vi "Final Line Detection System_2.vi"() -> ()   [LabVIEW 2017]
uses:
  <vilib>/userdefined/High Color/IMAQdx.ctl
  <vilib>/vision/driver/NI_Vision_Acquisition_Software.lvlib
  <vilib>/vision/NI_Vision_Development_Module.lvlib
panel:
  in  "Line Colour":string(combo)="Black"
  out "String 2":string
  in  "Maintenance":bool
  out "SpeechLib.ISpeechVoice 2":refnum<k7>
  in  "CHOOSE A VOICE:":i32(ring) items=["Microsoft Hazel Desktop - English (Great Britain)", "eSpeak-EN+M2", "eSpeak-EN-N"]
  in  "SpeechLib.ISpeechVoice":refnum<k7>
  out "Caution":bool
  out "Warning Message":string="Warning Obstacle!"
  out "Front IR Output voltage":dbl
  out "Back IR Output voltage":dbl
  out "Right IR Output voltage":dbl
  in  "Back IR Object Distance":dbl(knob)=80.0 min=0.0 max=100.0 step=1.0 scale=10.0..80.0
  in  "Front IR Object Distance":dbl(knob)=80.0 min=0.0 max=100.0 step=1.0 scale=10.0..80.0
  in  "Right IR Object Distance":dbl(knob)=80.0 min=0.0 max=100.0 step=1.0 scale=10.0..80.0
  out "error out 2":errorcluster
  out "Video Stream":T1(plugin-control)
  in  "stop":bool
  out "Found":bool
  out "error out 3":errorcluster
  out "error out 8":errorcluster
  out "error out 4":errorcluster
  in  "Barcode Types To Search":u32[](array[ring])=[6, 4] items=["Reserved", "Codabar", "Code 39", "Code 93", "Code 128", "EAN 8", "EAN 13", "Interleaved 2 of 5", "MSI", "UPCA", "Pharmacode", "RSS Limited"]
  out "error out 5":errorcluster
  in  "Select Vision System":string(combo)="None"
  out "Data":string
  in  "Recipients":string="chyslop@hotmail.co.uk, b8026896@my.shu.ac.uk,"
  in  "Subject":string
  in  "Message":string
  out "Primary IP Address":string
  out "All Other IP Addresses":string
  out "Number of Addresses":i32
  out "error out":errorcluster
  in  "Send":bool
  out "String":string
  in  "Session In":T2="cam1"
  in  "Noise IR Sensor 0 = no noise":dbl
  out "Left IR Output voltage":dbl
  in  "Left IR Object Distance":dbl(knob)=80.0 min=0.0 max=100.0 step=1.0 scale=10.0..80.0
  out "Right Motor Speedometer (m/s)":dbl(knob) scale=-2.5..2.5
  out "Left Motor Speedometer (m/s)":dbl(knob) scale=-2.5..2.5
  out "Right voltage more than 0?":bool
  out "Right Line sensor output voltage":dbl
  in  "Right Line Detector Sensor":dbl(slide) scale=0.0..5.0
  out "Left Voltage more than 0?":bool
  out "Left Line sensor output voltage":dbl
  in  "Left Line Detector Sensor":dbl(slide) scale=0.0..5.0
  out "Middle voltage more than 0?":bool
  out "Middle Line sensor output voltage":dbl
  in  "Middle Line Detector Sensor":dbl(slide) scale=0.0..5.0
  in  "Noise Line sensor, 0 = no noise":dbl
  in  "Stop":bool
  out "Direction":string
  out "Speedometer (m/s)":dbl(knob) scale=0.0..3.0
  in  "% Power":dbl(slide) scale=0.0..100.0
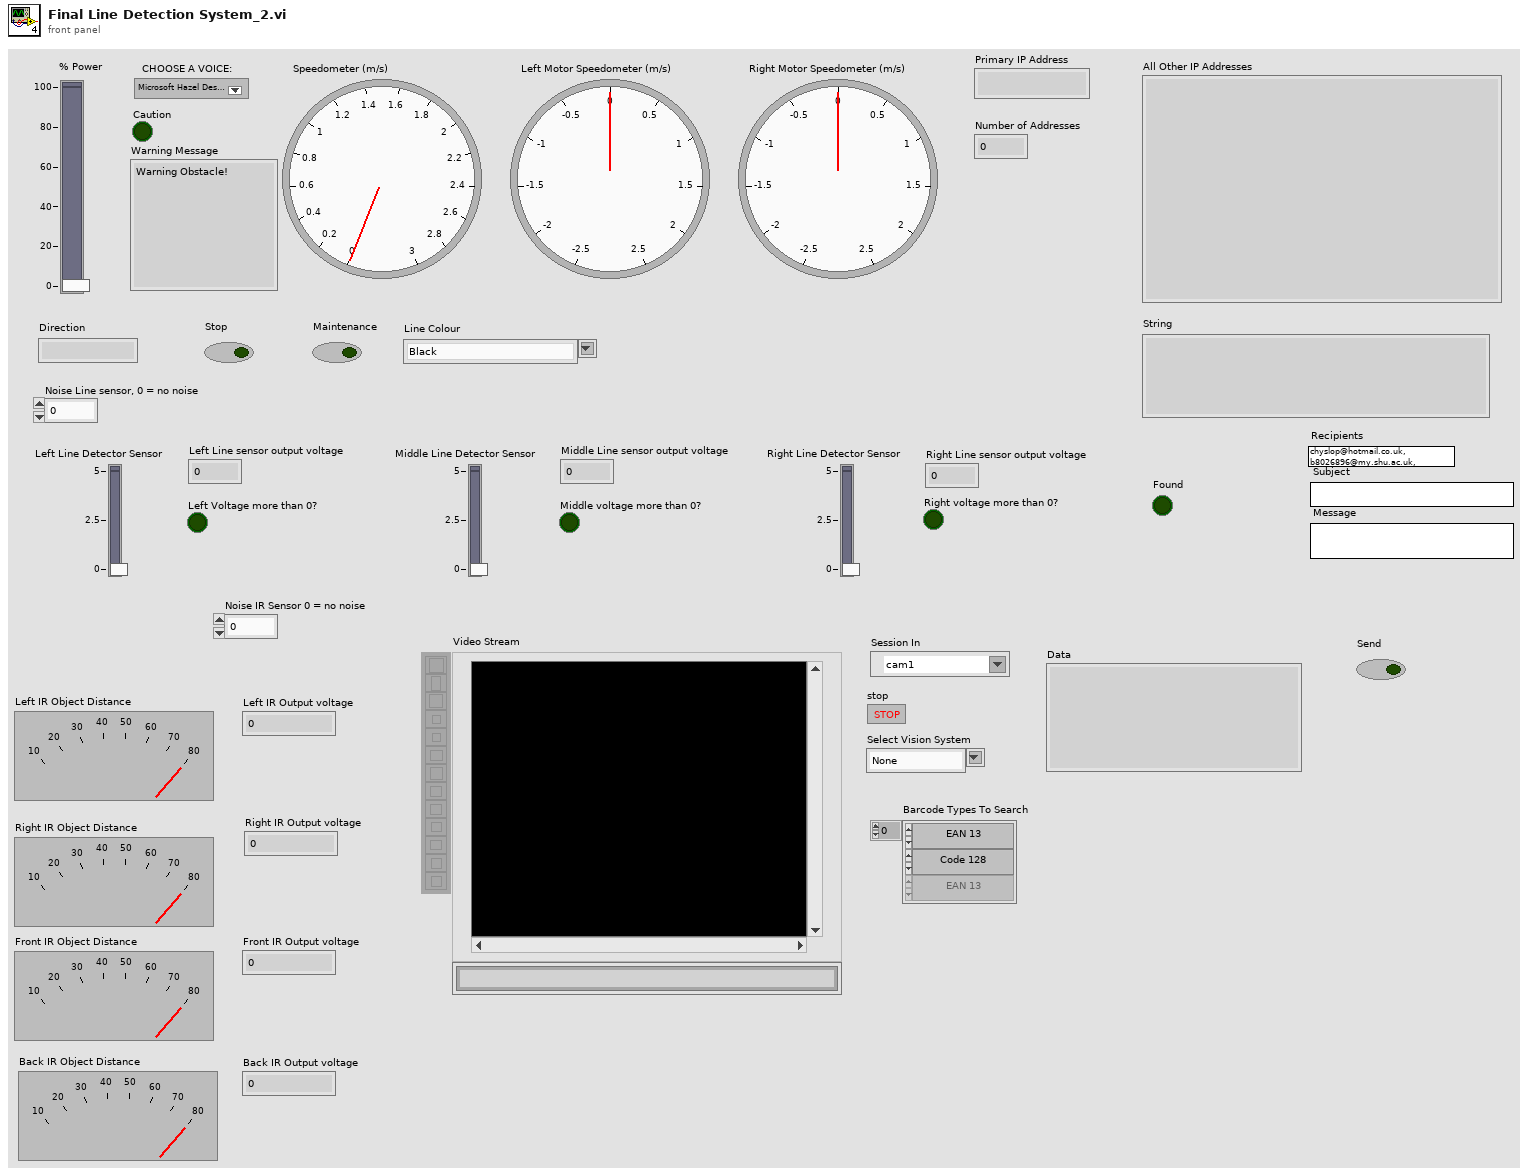
[diagram p1: front panel]
types:
  T1 = typedef "IMAQ Image.ctl" = refnum<image>
  T2 = typedef "IMAQdx.ctl" = refnum<k21>
  T3 = typedef "Image Type" = u32
  T4 = cluster{"Data":string, "Special Char 1":string, "Special Char 2":string, "Checksum(s)":string, "Barcode Type":u32, "Confidence Level":sgl, "Bounding Box":cluster{"x":sgl, "y":sgl}[]}[]
  T5 = cluster{"Data":string, "Special Char 1":string, "Special Char 2":string, "Checksum(s)":string, "Barcode Type":u32, "Confidence Level":sgl, "Bounding Box":cluster{"x":sgl, "y":sgl}[]}
  T6 = typedef "QR Code Report.ctl" = cluster{"Found?":bool, "Data":string, "Bounding Box":cluster{"x":sgl, "y":sgl}[], "Errors Corrected":u32, "Dimensions (Rows/Cols)":u32, "Version":u32, "QR Model":T7, "Stream Mode":T8, "Barcode Polarity":T9, "Mirrored?":bool, "Append Stream Position":u32, "Size of Append Stream":u32, "First EAN-128 ID":i32, "First Alternate Language ID":i32, "Append Stream ID":u32, "Minimum Edge Strength":u32, "Demodulation Mode":T10, "Cell Sample Size":T11, "Cell Filter Mode":T12}
  T7 = typedef "QR Code Model Type.ctl" = i32
  T8 = typedef "QR Code Stream Mode Type.ctl" = i32
  T9 = typedef "Data Matrix Polarity.ctl" = i32
  T10 = typedef "Demodulation Mode.ctl" = i32
  T11 = typedef "Cell Sample Size.ctl" = i32
  T12 = typedef "Cell Filter Mode.ctl" = i32
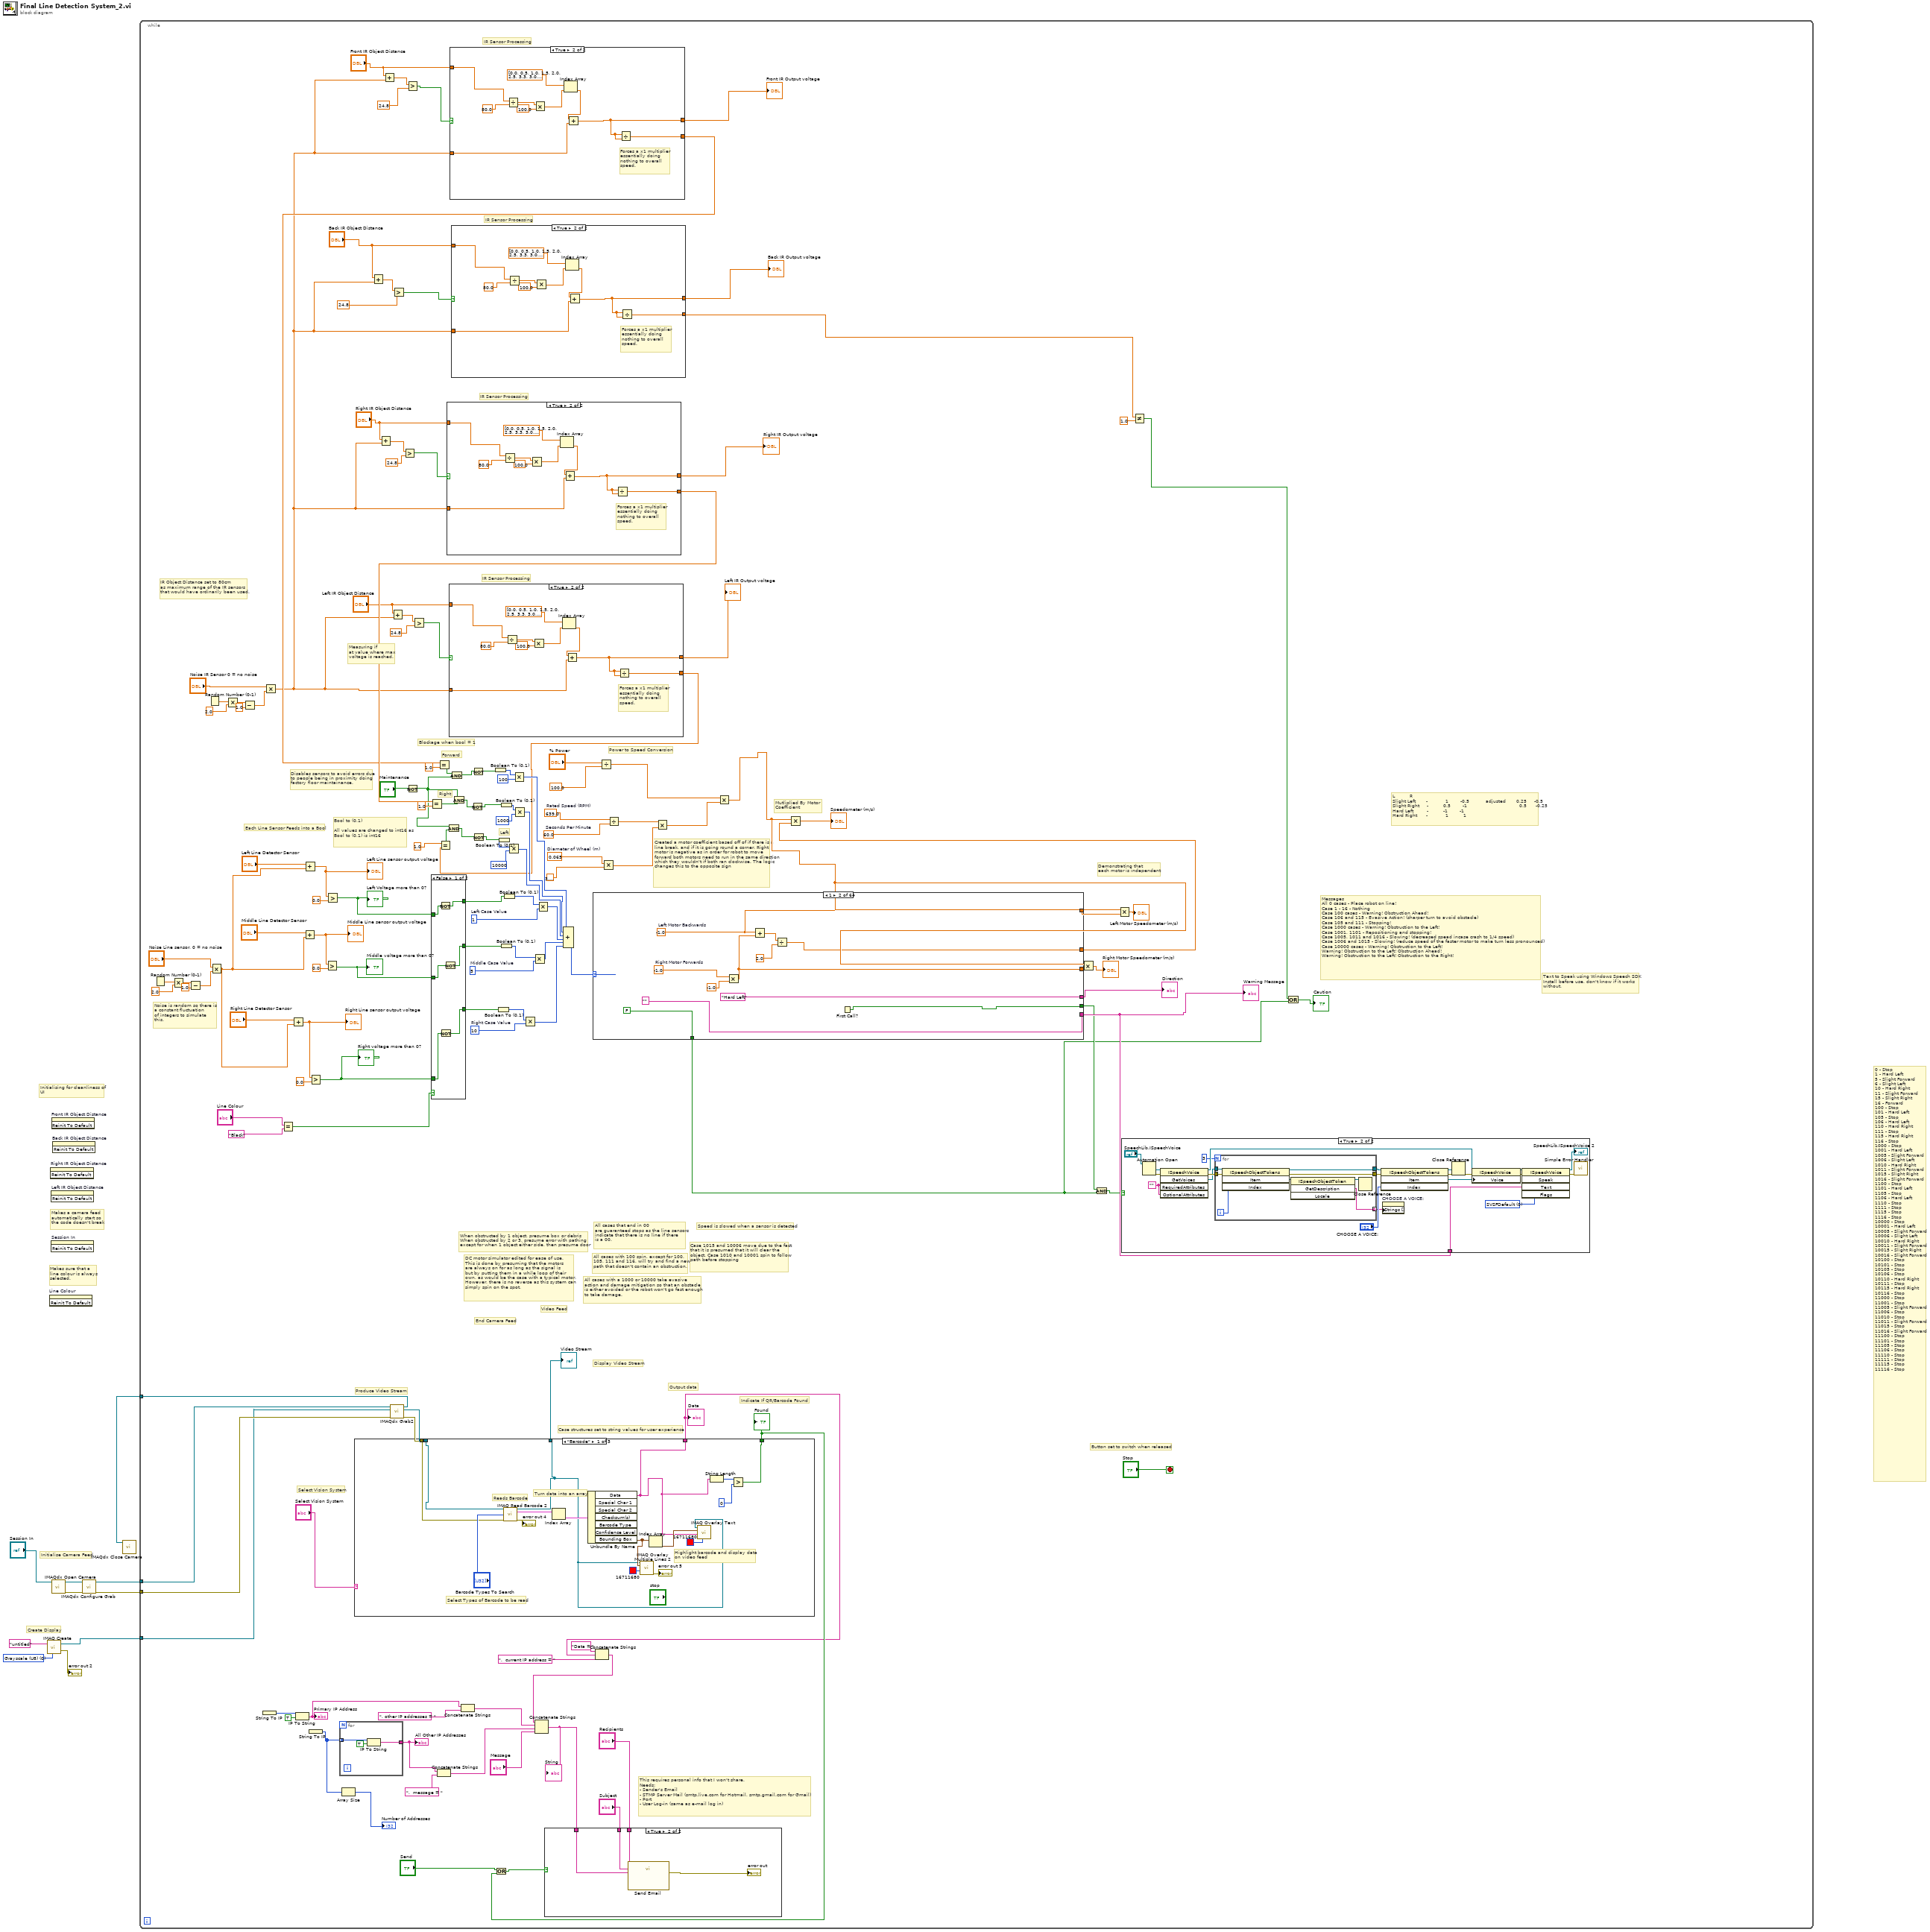
[diagram p0: block diagram]
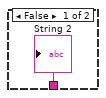
[diagram p3: hidden frame]
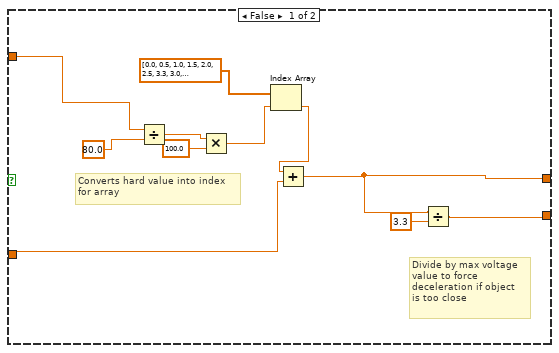
[diagram p4: hidden frame]
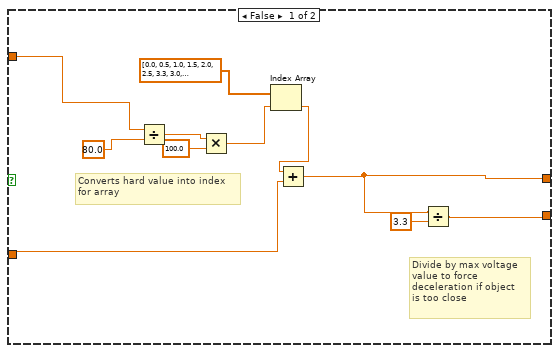
[diagram p5: hidden frame]
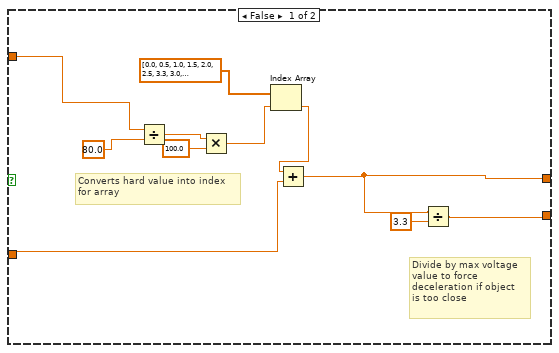
[diagram p6: hidden frame]
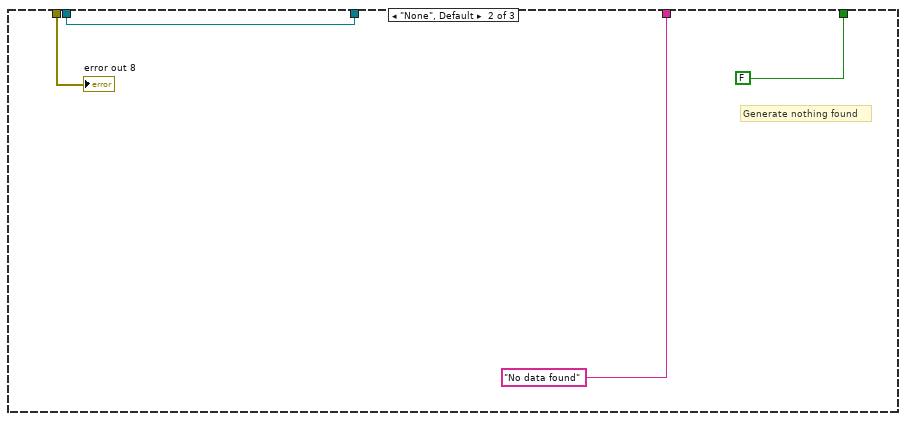
[diagram p8: hidden frame]
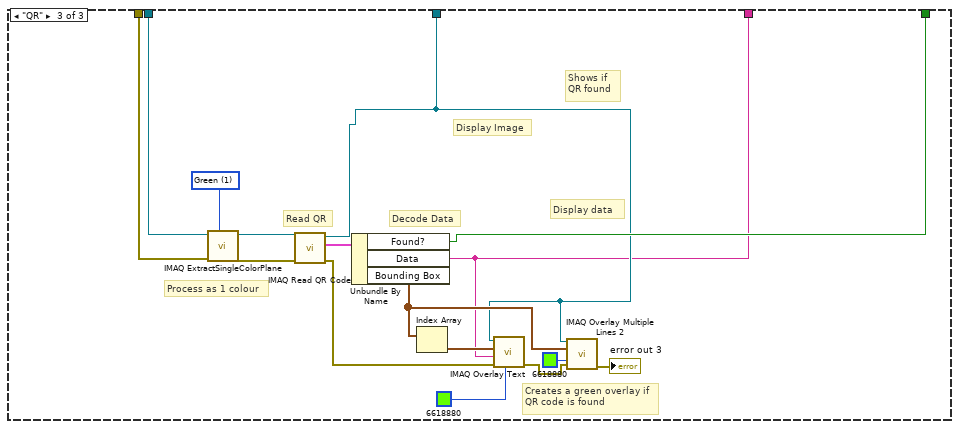
[diagram p9: hidden frame]
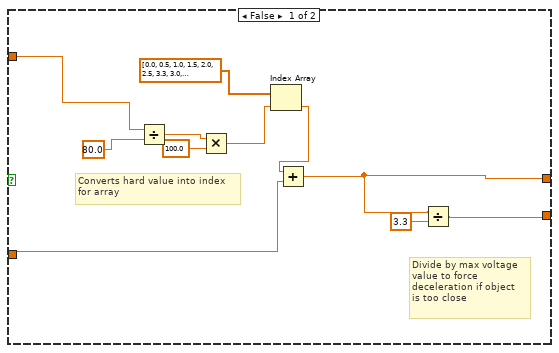
[diagram p10: hidden frame]
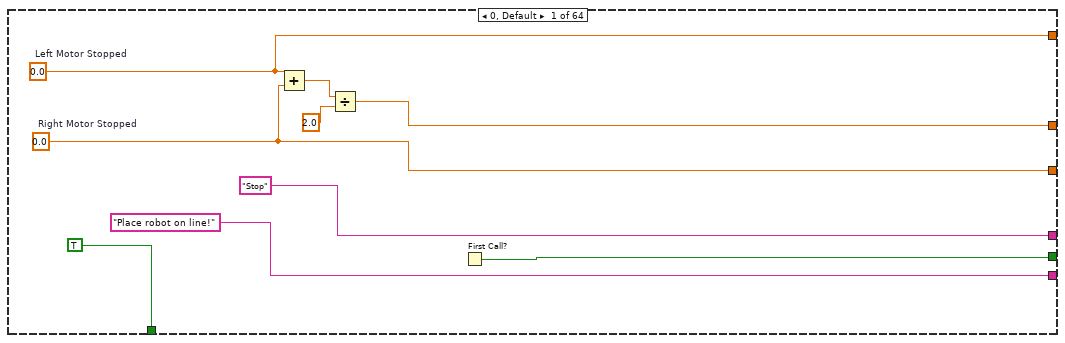
[diagram p11: hidden frame]
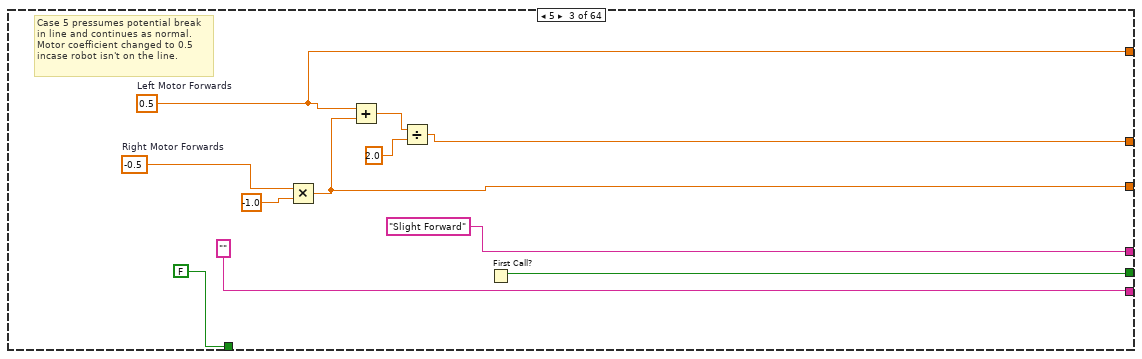
[diagram p12: hidden frame]
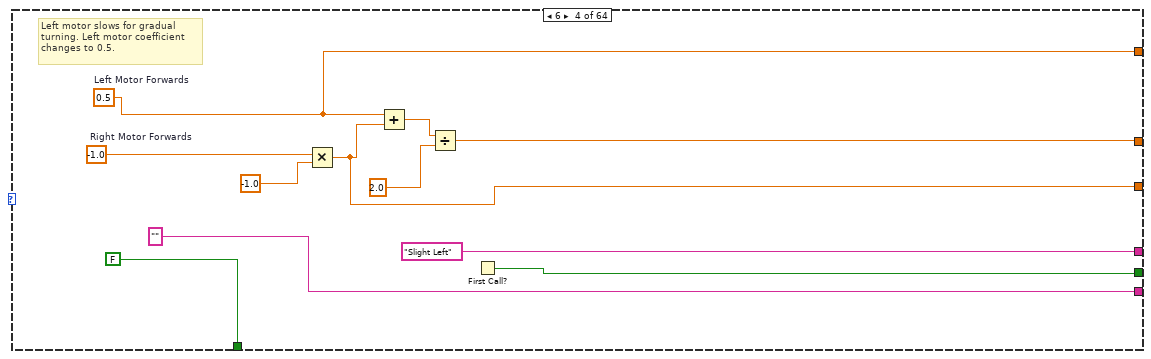
[diagram p13: hidden frame]
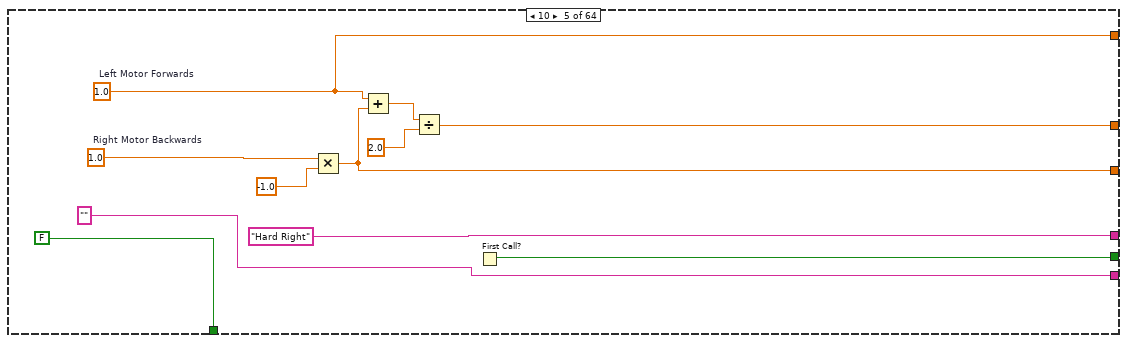
[diagram p14: hidden frame]
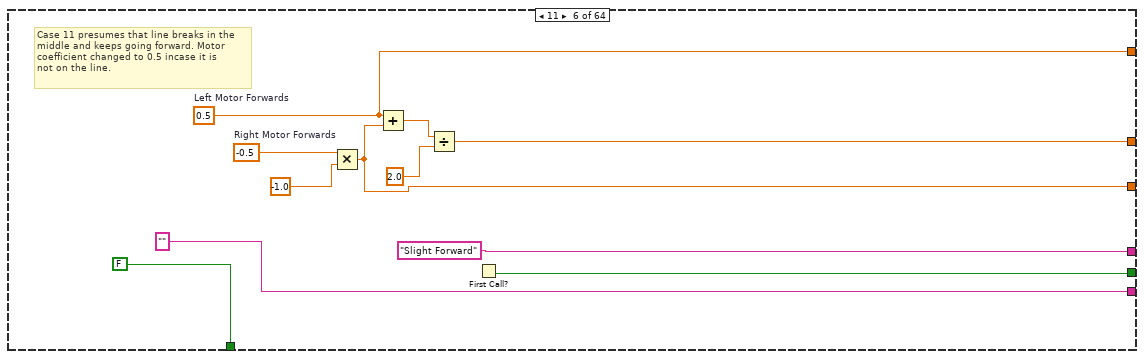
[diagram p15: hidden frame]
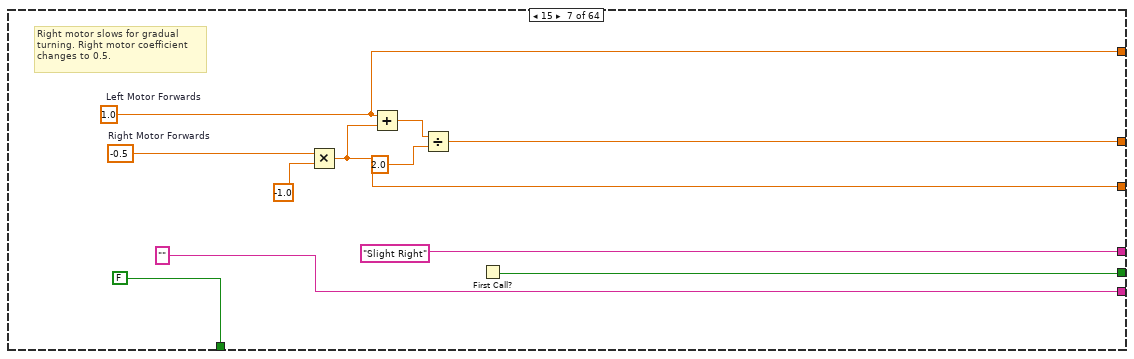
[diagram p16: hidden frame]
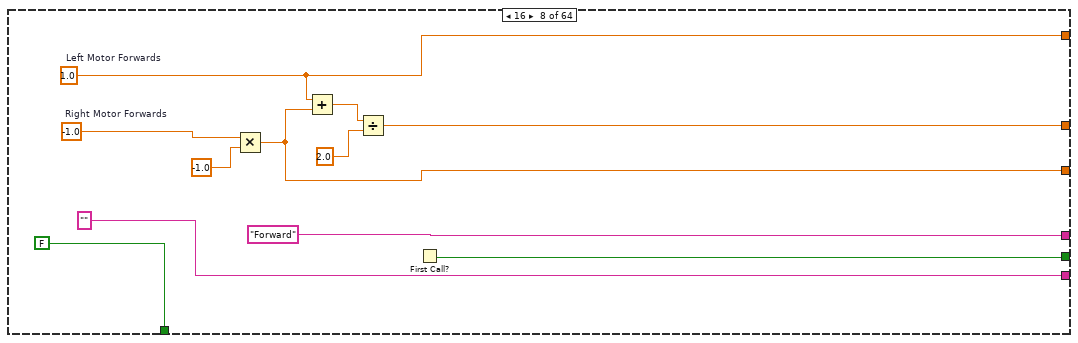
[diagram p17: hidden frame]
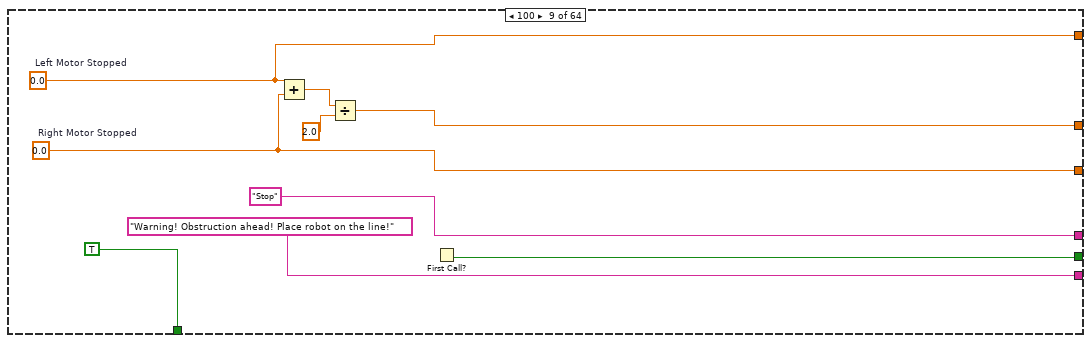
[diagram p18: hidden frame]
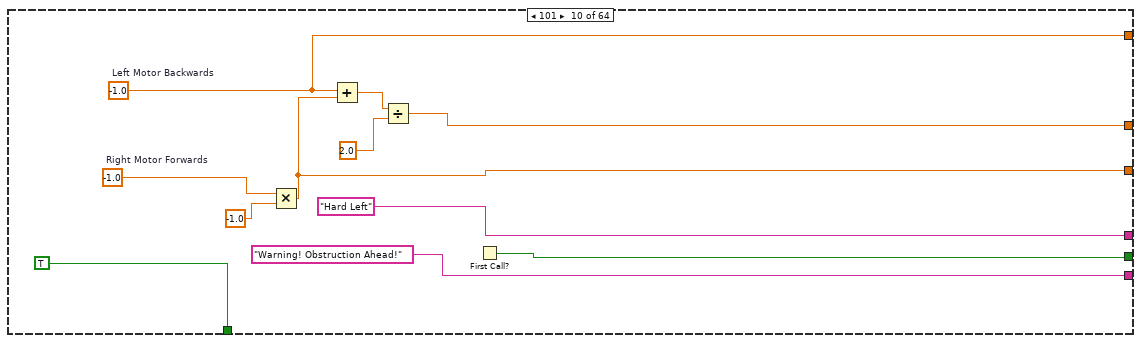
[diagram p19: hidden frame]
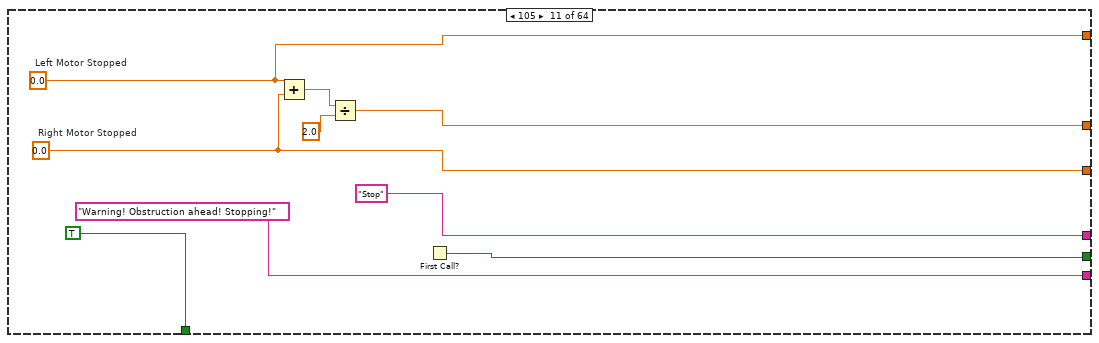
[diagram p20: hidden frame]
diagram:
  w5 = T3 0 items=["Grayscale (U8)", "Grayscale (I16)", "Grayscale (SGL)", "Complex (CSG)", "RGB (U32)", "HSL (U32)", "RGB (U64)", "Grayscale (U16)"] ("Image Type")
  # "Create Display"
  # "Initialise Camera Feed"
  # "Makes sure that a\nline colour is always\nselected."
  # "Initialising for cleanliness of\nUI"
  # "0 - Stop\n1 - Hard Left\n5 - Slight Forward\n6 - Slight Left\n10 - Hard Right\n11 - Slight Forward \n15 - Slight Right \n16 - Forward \n100 - Stop\n101 - Hard Left\n105 - Stop\n106 - Hard Left\n110 - Hard Right\n111 - Stop\n115 - Hard Right\n116 - Stop\n1000 - Stop\n1001 - Hard Left\n1005 - Slight Forward \n1006 - Slight Left \n1010 - Hard Right\n1011 - Slight Forward\n1015 - Slight Right\n1016 - Slight Forward\n1100 - Stop\n1101 - Hard Left\n1105 - Stop\n1106 - Hard Left\n1110 - Stop\n1111 - Stop\n1115 - Stop\n1116 - Stop\n10000 - Stop \n10001 - Hard Left \n10005 - Slight Forward\n10006 - Slight Left\n10010 - Hard Right\n10011 - Slight Forward\n10015 - Slight Right\n10016 - Slight Forward\n10100 - Stop\n10101 - Stop\n10105 - Stop\n10106 - Stop\n10110 - Hard Right\n10111 - Stop\n10115 - Hard Right\n10116 - Stop\n11000 - Stop \n11001 - Stop\n11005 - Slight Forward\n11006 - Stop\n11010 - Stop\n11011 - Slight Forward\n11015 - Stop\n11016 - Slight Forward\n11100 - Stop\n11101 - Stop\n11105 - Stop\n11106 - Stop\n11110 - Stop\n11111 - Stop\n11115 - Stop\n11116 - Stop"
  # "Makes a camera feed\nautomatically start so\nthe code doesn't break"
  n1 = call "IMAQ Create"("Image Name"="untitled", "Image Type"=w5) -> ("New Image"=w2:T1, "error out"=→"error out 2":errorcluster)  [unwired: 3 in]
  n2 = invoke on="Line Colour" class="CmbBox" method="Reinit To Default"() -> ()  [unwired: 3 in, 3 out]
  n3 = invoke on="Right IR Object Distance" class="Knob (strict)" method="Reinit To Default"() -> ()  [unwired: 3 in, 3 out]
  n4 = invoke on="Left IR Object Distance" class="Knob (strict)" method="Reinit To Default"() -> ()  [unwired: 3 in, 3 out]
  n5 = invoke on="Session In" class="IMAQdx (strict)" method="Reinit To Default"() -> ()  [unwired: 3 in, 3 out]
  n6 = invoke on="Front IR Object Distance" class="Knob (strict)" method="Reinit To Default"() -> ()  [unwired: 3 in, 3 out]
  n7 = call <vilib>:"IMAQdx Open Camera.vi"("Session In"="Session In") -> ("error out"=w8:errorcluster, "Session Out"=w7:T2)  [unwired: 9 in]
  n8 = invoke on="Back IR Object Distance" class="Knob (strict)" method="Reinit To Default"() -> ()  [unwired: 3 in, 3 out]
  n9 = call <vilib>:"IMAQdx Configure Grab.vi"("error in"=w8, "Session In"=w7) -> ("error out"=w4:errorcluster, "Session Out"=w3:T2)  [unwired: 8 in]
  n10 = while {
    tunnel: w4 -> [w27]
    tunnel: w3 -> [w26]
    tunnel: w2 -> [w25]
    tunnel: [w24] -> w1
    stop <- "Stop" stop-if-true
    w137 = i16 5  # Middle Case Value
    w132 = i16 10  # Right Case Value
    w136 = i16 1  # Left Case Value
    w151 = 0.065  # Diameter of Wheel (m)
    w152 = 60.0  # Seconds Per Minute
    w153 = 639.0  # Rated Speed (RPM)
    # "Text to Speak using Windows Speech SDK\nInstall before use, don't know if it works\nwithout."
    # "L          R\nSlight Left       -            1        -0.5           adjusted       0.25     -0.5     \nSlight Right     -          0.5        -1                                   0.5      -0.25\nHard Left         -          -1        -1       \nHard Right      -            1          1"
    # "Messages\nAll 0 cases - Place robot on line!\nCase 1 - 16 - Nothing\nCase 100 cases - Warning! Obstruction Ahead!\nCase 106 and 115 - Evasive Action! (sharper turn to avoid obstacle)\nCase 105 and 111 - Stopping!\nCase 1000 cases - Warning! Obstruction to the Left!\nCase 1001, 1101 - Repositioning and stopping!\nCase 1005, 1011 and 1016 - Slowing! (decreased spead incase crash to 1/4 speed)\nCase 1006 and 1015 - Slowing! (reduce speed of the faster motor to make turn less pronounced) \nCase 10000 cases - Warning! Obstruction to the Left!\nWarning! Obstruction to the Left! Obstruction Ahead!\nWarning! Obstruction to the Left! Obstruction to the Right!"
    # "Case 1015 and 10006 move due to the fact that it is presumed that it will clear the object. Case 1010 and 10001 spin to follow path before stopping"
    # "Speed is slowed when a sensor is detected"
    # "Disables sensors to avoid errors due\nto people being in proximity doing\nfactory floor maintainance."
    # "When obstructed by 1 object, presume box or debris\nWhen obstructed by 2 or 3, presume error with pathing\nexcept for when 1 object either side, then presume door"
    # "All cases with a 1000 or 10000 take evasive\naction and damage mitigation so that an obstacle\nis either avoided or the robot won't go fast enough\nto take damage."
    # "All cases with 100 spin, except for 100,\n105, 111 and 116, will try and find a new\npath that doesn't contain an obstruction."
    # "All cases that end in 00\nare guaranteed stops as the line sensors\nindicate that there is no line if there\nis a 00."
    # "Blockage when bool = 1"
    # "Forward"
    # "Right"
    # "Left"
    # "IR Sensor Processing"
    # "IR Sensor Processing"
    # "IR Sensor Processing"
    # "This requires personal info that I won't share.\nNeeds:\n- Sender's Email\n- STMP Server Mail (smtp.live.com for Hotmail, smtp.gmail.com for Gmail)\n- Port\n- User Log-in (same as e-mail log in)"
    # "Output data"
    # "Case structures set to string values for user experience"
    # "Select Vision System"
    # "Indicate If QR/Barcode Found"
    # "Display Video Stream"
    # "Produce Video Stream"
    # "Video Feed"
    # "End Camera Feed"
    # "IR Object Distance set to 80cm\nas maximum range of the IR sensors\nthat would have ordinarily been used."
    # "Measuring if\nat value where max\nvoltage is reached."
    # "IR Sensor Processing"
    # "Demonstrating that\neach motor is independent"
    # "DC motor simulator edited for ease of use.\nThis is done by presuming that the motors\nare always on for as long as the signal is\nbut by putting them in a while loop of their\nown, as would be the case with a typical motor.\nHowever, there is no reverse as this system can\nsimply spin on the spot."
    # "Noise is random so there is\na constant fluctuation\nof integers to simulate\nthis."
    # "Each Line Sensor Feeds into a Bool"
    # "Created a motor coefficient based off of if there is a line break, and if it is going round a corner. Right motor is negative as in order for robot to move forward both motors need to run in the same direction which they wouldn't if both ran clockwise. The logic changes this to the opposite sign"
    # "Mutliplied By Motor\nCoefficient"
    # "Button set to switch when released"
    # "Bool to (0,1)\n\nAll values are changed to int16 as Bool to (0,1) is int16"
    # "Power to Speed Conversion"
    n11 = Random Number (0-1)() -> (number: 0 to 1=w120:dbl)
    n12 = Multiply(x=w120, y=2.0) -> (x*y=w119:dbl)
    n13 = Subtract(x=w119, y=1.0) -> (x-y=w118:dbl)
    n14 = Random Number (0-1)() -> (number: 0 to 1=w105:dbl)
    n15 = Multiply(x="Noise Line sensor, 0 = no noise", y=w118) -> (x*y=w115:dbl)
    n16 = Multiply(x=w105, y=2.0) -> (x*y=w106:dbl)
    n17 = Subtract(x=w106, y=1.0) -> (x-y=w107:dbl)
    n18 = String To IP() -> (0:w97:u32)  [unwired: 1 in]
    n19 = Multiply(x="Noise IR Sensor 0 = no noise", y=w107) -> (x*y=w30:dbl)
    n20 = Equal?(x="Line Colour", y="Black") -> (x = y?=w11:bool)
    n21 = Add(x="Right Line Detector Sensor", y=w115) -> (x+y=w123:dbl)
    "Right Line sensor output voltage" <- w123
    n22 = IP To String(1:TRUE ("dot notation? (F)"), 2:w97) -> (0:w84:string)
    "Primary IP Address" <- w84
    n23 = Add(x="Middle Line Detector Sensor", y=w115) -> (x+y=w129:dbl)
    "Middle Line sensor output voltage" <- w129
    n24 = Add(x="Left Line Detector Sensor", y=w115) -> (x+y=w126:dbl)
    "Left Line sensor output voltage" <- w126
    n25 = String To IP() -> (0:w96:u32[])  [unwired: 1 in]
    n26 = Greater?(x=w123, y=0.0) -> (0:w13:bool)
    "Right voltage more than 0?" <- w13
    n27 = Greater?(x=w129, y=0.0) -> (0:w14:bool)
    "Middle voltage more than 0?" <- w14
    n28 = Greater?(x=w126, y=0.0) -> (0:w16:bool)
    "Left Voltage more than 0?" <- w16
    n29 = for {
      tunnel: w96 -> [w264] mode=indexing
      tunnel: [w262] -> w80
      n30 = IP To String(1:TRUE ("dot notation? (F)"), 2:w264) -> (0:w262:string)
    }
    "All Other IP Addresses" <- w80
    n31 = Array Size(array=w96) -> (size(s)=→"Number of Addresses":i32)
    n32 = Add(x="Back IR Object Distance", y=w30) -> (x+y=w37:dbl)
    n33 = Add(x="Right IR Object Distance", y=w30) -> (x+y=w35:dbl)
    n34 = Add(x="Front IR Object Distance", y=w30) -> (x+y=w39:dbl)
    n35 = call <vilib>:"IMAQdx Grab2.vi"("error in"=w27, "Image In"=w25, "Session In"=w26) -> ("error out"=w98:errorcluster, "Image Out"=w101:T1, "Session Out"=w24:T2)  [unwired: 5 in, 1 out]
    n36 = case shown="\"Barcode\"" "Select Vision System" {
      tunnel: w101 -> [w268 w283 w287]
      tunnel: w98 -> [w267 w284 w286]
      tunnel: [w266 FALSE w289] -> w87
      tunnel: [w269 w283 w288] -> w100
      tunnel: [w265 "No data found" w285] -> w78
      frame "Barcode" {
        # "Highlight barcode and display data\non video feed"
        # "Turn data into an array"
        # "Select Types of Barcode to be read"
        # "Reads Barcode"
        n37 = call "IMAQ Read Barcode 2"("Image"=w268, "Barcode Types To Search"="Barcode Types To Search", "error in (no error)"=w267) -> ("Image (duplicate)"=w269:T1, "Barcodes"=w275:T4, "error out"=→"error out 4":errorcluster)  [unwired: 8 in, 2 out]
        n38 = Index Array(array=w275) -> (element=w276:T5)  [unwired: 1 in]
        n39 = Unbundle By Name(w276) -> ("Data"=w265:string, "Bounding Box"=w278:cluster{"x":sgl, "y":sgl}[])  [unwired: 5 out]
        n40 = call "IMAQ Overlay Multiple Lines 2"("Image"=w269, "Line End Points"=w278, "Color"=u32 16711680) -> ("error out"=→"error out 5":errorcluster)  [unwired: 11 in, 1 out]
        n41 = Index Array(array=w278) -> (element=w277:cluster{"x":sgl, "y":sgl})  [unwired: 1 in]
        n42 = call "IMAQ Overlay Text"("Text Color (black)"=u32 16711680, "String"=w265, "Origin"=w277, "Image"=w269) -> ()  [unwired: 6 in, 2 out]
        n43 = String Length(string=w265) -> (length=w280:i32)
        n44 = Greater?(x=w280, y=0) -> (0:w266:bool)
      }
      frame "None", Default {
        # "Generate nothing found"
        "error out 8" <- w284
      }
      frame "QR" {
        w298 = 1 items=["Red", "Green", "Blue", "Hue", "Saturation", "Luminance", "Value", "Intensity"] ("Color Plane")
        # "Creates a green overlay if\nQR code is found"
        # "Shows if\nQR found"
        # "Display data"
        # "Decode Data"
        # "Display Image"
        # "Read QR"
        # "Process as 1 colour"
        n45 = call "IMAQ ExtractSingleColorPlane"("Color Plane"=w298, "error in (no error)"=w286, "Image Src"=w287) -> ("error out"=w299:errorcluster, "Image Dst Out"=w300:T1)  [unwired: 7 in]
        n46 = call "IMAQ Read QR Code"("error in (no error)"=w299, "Image"=w300) -> ("error out"=w290:errorcluster, "QR Code Report"=w297:T6, "Image (duplicate)"=w288:T1)  [unwired: 6 in, 1 out]
        n47 = Unbundle By Name(w297) -> ("Found?"=w289:bool, "Data"=w285:string, "Bounding Box"=w294:cluster{"x":sgl, "y":sgl}[])
        n48 = Index Array(array=w294) -> (element=w296:cluster{"x":sgl, "y":sgl})  [unwired: 1 in]
        n49 = call "IMAQ Overlay Text"("Text Color (black)"=u32 6618880, "error in (no error)"=w290, "String"=w285, "Origin"=w296, "Image"=w288) -> ("error out"=w292:errorcluster)  [unwired: 5 in, 1 out]
        n50 = call "IMAQ Overlay Multiple Lines 2"("Image"=w288, "Line End Points"=w294, "Color"=u32 6618880, "error in (no error)"=w292) -> ("error out"=→"error out 3":errorcluster)  [unwired: 10 in, 1 out]
      }
    }
    "Video Stream" <- w100
    "Found" <- w87
    "Data" <- w78
    n51 = Add(x="Left IR Object Distance", y=w30) -> (x+y=w32:dbl)
    n52 = Greater?(x=w37, y=24.8) -> (0:w72:bool)
    n53 = Greater?(x=w35, y=24.8) -> (0:w71:bool)
    n54 = Greater?(x=w39, y=24.8) -> (0:w73:bool)
    n55 = Not(x="Maintenance") -> (.not. x?=w53:bool)
    n56 = Greater?(x=w32, y=24.8) -> (0:w102:bool)
    n57 = case shown="False" w11 {
      tunnel: [w159 w163] -> w17
      tunnel: w16 -> [w160 w163]
      tunnel: [w158 w162] -> w15
      tunnel: w14 -> [w157 w162]
      tunnel: w13 -> [w155 w161]
      tunnel: [w156 w161] -> w12
      frame False {
        n58 = Not(x=w160) -> (.not. x?=w159:bool)
        n59 = Not(x=w155) -> (.not. x?=w156:bool)
        n60 = Not(x=w157) -> (.not. x?=w158:bool)
      }
      frame True {
      }
    }
    n61 = Concatenate Strings(w80, ",  message = " ("string")) -> (w81:string)
    n62 = case shown="True" w71 {
      tunnel: "Right IR Object Distance" -> [w241 w257]
      tunnel: [w238 w250] -> w76
      tunnel: [w239 w249] -> w68
      tunnel: w30 -> [w240 w248]
      frame False {
        # "Converts hard value into index\nfor array"
        # "Divide by max voltage\nvalue to force\ndeceleration if object\nis too close"
        n63 = Divide(x=w241, y=80.0) -> (x/y=w246:dbl)
        n64 = Multiply(x=w246, y=100.0) -> (x*y=w247:dbl)
        n65 = Index Array(array=dbl[] [0.0, 0.5, 1.0, 1.5, 2.0, 2.5, 3.3, 3.0, 2.658255897, 2.408413052, 2.20488628, 2.035631323, 1.892484412, 1.769708211, 1.663148013, 1.569718295, 1.487077661, 1.413415986, 1.347310939, 1.287628787, 1.233454287, 1.184040141, 1.138769924, 1.097130449, 1.058690886, 1.023086768, 0.990007602, 0.959187169, 0.930395851, 0.903434503, 0.878129533, 0.854328896, 0.83189883, 0.81072117, 0.790691122, 0.771715412, 0.753710732, 0.736602435, 0.72032343, 0.704813241, 0.690017209, 0.675885801, 0.66237402, 0.64944089, 0.63704902, 0.625164212, 0.613755126, 0.602792986, 0.592251321, 0.582105738, 0.572333717, 0.562914438, 0.553828618, 0.545058374, 0.536587096, 0.528399334, 0.520480698, 0.51281777, 0.50539802, 0.498209735, 0.491241951, 0.484484395, 0.477927433, 0.471562015, 0.465379637, 0.459372298, 0.453532462, 0.447853023, 0.442327281, 0.436948907, 0.431711917, 0.426610656, 0.421639765, 0.416794173, 0.412069067, 0.407459883, 0.402962289, 0.398572167, 0.394285602, 0.39009887, 0.386008427, 0.382010895, 0.378103055, 0.374281838, 0.370544314, 0.366887686, 0.363309281, 0.359806547, 0.35637704, 0.353018422, 0.349728457, 0.346505002, 0.343346003, 0.340249491, 0.337213578, 0.334236453, 0.331316376, 0.328451676, 0.325640748, 0.32288205, 0.320174098] ("first row"), index=w247) -> (element=w245:dbl)
        n66 = Add(x=w245, y=w240) -> (x+y=w238:dbl)
        n67 = Divide(x=w238, y=3.3) -> (x/y=w239:dbl)
      }
      frame True {
        # "Forces a x1 multiplier\nessentially doing\nnothing to overall\nspeed."
        n68 = Divide(x=w257, y=80.0) -> (x/y=w255:dbl)
        n69 = Multiply(x=w255, y=100.0) -> (x*y=w256:dbl)
        n70 = Index Array(array=dbl[] [0.0, 0.5, 1.0, 1.5, 2.0, 2.5, 3.3, 3.0, 2.658255897, 2.408413052, 2.20488628, 2.035631323, 1.892484412, 1.769708211, 1.663148013, 1.569718295, 1.487077661, 1.413415986, 1.347310939, 1.287628787, 1.233454287, 1.184040141, 1.138769924, 1.097130449, 1.058690886, 1.023086768, 0.990007602, 0.959187169, 0.930395851, 0.903434503, 0.878129533, 0.854328896, 0.83189883, 0.81072117, 0.790691122, 0.771715412, 0.753710732, 0.736602435, 0.72032343, 0.704813241, 0.690017209, 0.675885801, 0.66237402, 0.64944089, 0.63704902, 0.625164212, 0.613755126, 0.602792986, 0.592251321, 0.582105738, 0.572333717, 0.562914438, 0.553828618, 0.545058374, 0.536587096, 0.528399334, 0.520480698, 0.51281777, 0.50539802, 0.498209735, 0.491241951, 0.484484395, 0.477927433, 0.471562015, 0.465379637, 0.459372298, 0.453532462, 0.447853023, 0.442327281, 0.436948907, 0.431711917, 0.426610656, 0.421639765, 0.416794173, 0.412069067, 0.407459883, 0.402962289, 0.398572167, 0.394285602, 0.39009887, 0.386008427, 0.382010895, 0.378103055, 0.374281838, 0.370544314, 0.366887686, 0.363309281, 0.359806547, 0.35637704, 0.353018422, 0.349728457, 0.346505002, 0.343346003, 0.340249491, 0.337213578, 0.334236453, 0.331316376, 0.328451676, 0.325640748, 0.32288205, 0.320174098] ("first row"), index=w256) -> (element=w254:dbl)
        n71 = Add(x=w254, y=w248) -> (x+y=w250:dbl)
        n72 = Divide(x=w250, y=w250) -> (x/y=w249:dbl)
      }
    }
    "Right IR Output voltage" <- w76
    n73 = Equal?(x=w68, y=1.0) -> (x = y?=w54:bool)
    n74 = case shown="True" w102 {
      tunnel: "Left IR Object Distance" -> [w305 w321]
      tunnel: [w302 w314] -> w110
      tunnel: [w303 w313] -> w29
      tunnel: w30 -> [w304 w312]
      frame False {
        # "Converts hard value into index\nfor array"
        # "Divide by max voltage\nvalue to force\ndeceleration if object\nis too close"
        n75 = Divide(x=w305, y=80.0) -> (x/y=w310:dbl)
        n76 = Multiply(x=w310, y=100.0) -> (x*y=w311:dbl)
        n77 = Index Array(array=dbl[] [0.0, 0.5, 1.0, 1.5, 2.0, 2.5, 3.3, 3.0, 2.658255897, 2.408413052, 2.20488628, 2.035631323, 1.892484412, 1.769708211, 1.663148013, 1.569718295, 1.487077661, 1.413415986, 1.347310939, 1.287628787, 1.233454287, 1.184040141, 1.138769924, 1.097130449, 1.058690886, 1.023086768, 0.990007602, 0.959187169, 0.930395851, 0.903434503, 0.878129533, 0.854328896, 0.83189883, 0.81072117, 0.790691122, 0.771715412, 0.753710732, 0.736602435, 0.72032343, 0.704813241, 0.690017209, 0.675885801, 0.66237402, 0.64944089, 0.63704902, 0.625164212, 0.613755126, 0.602792986, 0.592251321, 0.582105738, 0.572333717, 0.562914438, 0.553828618, 0.545058374, 0.536587096, 0.528399334, 0.520480698, 0.51281777, 0.50539802, 0.498209735, 0.491241951, 0.484484395, 0.477927433, 0.471562015, 0.465379637, 0.459372298, 0.453532462, 0.447853023, 0.442327281, 0.436948907, 0.431711917, 0.426610656, 0.421639765, 0.416794173, 0.412069067, 0.407459883, 0.402962289, 0.398572167, 0.394285602, 0.39009887, 0.386008427, 0.382010895, 0.378103055, 0.374281838, 0.370544314, 0.366887686, 0.363309281, 0.359806547, 0.35637704, 0.353018422, 0.349728457, 0.346505002, 0.343346003, 0.340249491, 0.337213578, 0.334236453, 0.331316376, 0.328451676, 0.325640748, 0.32288205, 0.320174098] ("first row"), index=w311) -> (element=w309:dbl)
        n78 = Add(x=w309, y=w304) -> (x+y=w302:dbl)
        n79 = Divide(x=w302, y=3.3) -> (x/y=w303:dbl)
      }
      frame True {
        # "Forces a x1 multiplier\nessentially doing\nnothing to overall\nspeed."
        n80 = Divide(x=w321, y=80.0) -> (x/y=w319:dbl)
        n81 = Multiply(x=w319, y=100.0) -> (x*y=w320:dbl)
        n82 = Index Array(array=dbl[] [0.0, 0.5, 1.0, 1.5, 2.0, 2.5, 3.3, 3.0, 2.658255897, 2.408413052, 2.20488628, 2.035631323, 1.892484412, 1.769708211, 1.663148013, 1.569718295, 1.487077661, 1.413415986, 1.347310939, 1.287628787, 1.233454287, 1.184040141, 1.138769924, 1.097130449, 1.058690886, 1.023086768, 0.990007602, 0.959187169, 0.930395851, 0.903434503, 0.878129533, 0.854328896, 0.83189883, 0.81072117, 0.790691122, 0.771715412, 0.753710732, 0.736602435, 0.72032343, 0.704813241, 0.690017209, 0.675885801, 0.66237402, 0.64944089, 0.63704902, 0.625164212, 0.613755126, 0.602792986, 0.592251321, 0.582105738, 0.572333717, 0.562914438, 0.553828618, 0.545058374, 0.536587096, 0.528399334, 0.520480698, 0.51281777, 0.50539802, 0.498209735, 0.491241951, 0.484484395, 0.477927433, 0.471562015, 0.465379637, 0.459372298, 0.453532462, 0.447853023, 0.442327281, 0.436948907, 0.431711917, 0.426610656, 0.421639765, 0.416794173, 0.412069067, 0.407459883, 0.402962289, 0.398572167, 0.394285602, 0.39009887, 0.386008427, 0.382010895, 0.378103055, 0.374281838, 0.370544314, 0.366887686, 0.363309281, 0.359806547, 0.35637704, 0.353018422, 0.349728457, 0.346505002, 0.343346003, 0.340249491, 0.337213578, 0.334236453, 0.331316376, 0.328451676, 0.325640748, 0.32288205, 0.320174098] ("first row"), index=w320) -> (element=w318:dbl)
        n83 = Add(x=w318, y=w312) -> (x+y=w314:dbl)
        n84 = Divide(x=w314, y=w314) -> (x/y=w313:dbl)
      }
    }
    "Left IR Output voltage" <- w110
    n85 = Equal?(x=1.0 ("y"), y=w29) -> (x = y?=w55:bool)
    n86 = And(x=w53, y=w55) -> (x .and. y?=w18:bool)
    n87 = case shown="True" w73 {
      tunnel: "Front IR Object Distance" -> [w199 w215]
      tunnel: [w196 w208] -> w74
      tunnel: [w197 w207] -> w67
      tunnel: w30 -> [w198 w206]
      frame False {
        # "Converts hard value into index\nfor array"
        # "Divide by max voltage\nvalue to force\ndeceleration if object\nis too close"
        n88 = Divide(x=w199, y=80.0) -> (x/y=w204:dbl)
        n89 = Multiply(x=w204, y=100.0) -> (x*y=w205:dbl)
        n90 = Index Array(array=dbl[] [0.0, 0.5, 1.0, 1.5, 2.0, 2.5, 3.3, 3.0, 2.658255897, 2.408413052, 2.20488628, 2.035631323, 1.892484412, 1.769708211, 1.663148013, 1.569718295, 1.487077661, 1.413415986, 1.347310939, 1.287628787, 1.233454287, 1.184040141, 1.138769924, 1.097130449, 1.058690886, 1.023086768, 0.990007602, 0.959187169, 0.930395851, 0.903434503, 0.878129533, 0.854328896, 0.83189883, 0.81072117, 0.790691122, 0.771715412, 0.753710732, 0.736602435, 0.72032343, 0.704813241, 0.690017209, 0.675885801, 0.66237402, 0.64944089, 0.63704902, 0.625164212, 0.613755126, 0.602792986, 0.592251321, 0.582105738, 0.572333717, 0.562914438, 0.553828618, 0.545058374, 0.536587096, 0.528399334, 0.520480698, 0.51281777, 0.50539802, 0.498209735, 0.491241951, 0.484484395, 0.477927433, 0.471562015, 0.465379637, 0.459372298, 0.453532462, 0.447853023, 0.442327281, 0.436948907, 0.431711917, 0.426610656, 0.421639765, 0.416794173, 0.412069067, 0.407459883, 0.402962289, 0.398572167, 0.394285602, 0.39009887, 0.386008427, 0.382010895, 0.378103055, 0.374281838, 0.370544314, 0.366887686, 0.363309281, 0.359806547, 0.35637704, 0.353018422, 0.349728457, 0.346505002, 0.343346003, 0.340249491, 0.337213578, 0.334236453, 0.331316376, 0.328451676, 0.325640748, 0.32288205, 0.320174098] ("first row"), index=w205) -> (element=w203:dbl)
        n91 = Add(x=w203, y=w198) -> (x+y=w196:dbl)
        n92 = Divide(x=w196, y=3.3) -> (x/y=w197:dbl)
      }
      frame True {
        # "Forces a x1 multiplier\nessentially doing\nnothing to overall\nspeed."
        n93 = Divide(x=w215, y=80.0) -> (x/y=w213:dbl)
        n94 = Multiply(x=w213, y=100.0) -> (x*y=w214:dbl)
        n95 = Index Array(array=dbl[] [0.0, 0.5, 1.0, 1.5, 2.0, 2.5, 3.3, 3.0, 2.658255897, 2.408413052, 2.20488628, 2.035631323, 1.892484412, 1.769708211, 1.663148013, 1.569718295, 1.487077661, 1.413415986, 1.347310939, 1.287628787, 1.233454287, 1.184040141, 1.138769924, 1.097130449, 1.058690886, 1.023086768, 0.990007602, 0.959187169, 0.930395851, 0.903434503, 0.878129533, 0.854328896, 0.83189883, 0.81072117, 0.790691122, 0.771715412, 0.753710732, 0.736602435, 0.72032343, 0.704813241, 0.690017209, 0.675885801, 0.66237402, 0.64944089, 0.63704902, 0.625164212, 0.613755126, 0.602792986, 0.592251321, 0.582105738, 0.572333717, 0.562914438, 0.553828618, 0.545058374, 0.536587096, 0.528399334, 0.520480698, 0.51281777, 0.50539802, 0.498209735, 0.491241951, 0.484484395, 0.477927433, 0.471562015, 0.465379637, 0.459372298, 0.453532462, 0.447853023, 0.442327281, 0.436948907, 0.431711917, 0.426610656, 0.421639765, 0.416794173, 0.412069067, 0.407459883, 0.402962289, 0.398572167, 0.394285602, 0.39009887, 0.386008427, 0.382010895, 0.378103055, 0.374281838, 0.370544314, 0.366887686, 0.363309281, 0.359806547, 0.35637704, 0.353018422, 0.349728457, 0.346505002, 0.343346003, 0.340249491, 0.337213578, 0.334236453, 0.331316376, 0.328451676, 0.325640748, 0.32288205, 0.320174098] ("first row"), index=w214) -> (element=w212:dbl)
        n96 = Add(x=w212, y=w206) -> (x+y=w208:dbl)
        n97 = Divide(x=w208, y=w208) -> (x/y=w207:dbl)
      }
    }
    "Front IR Output voltage" <- w74
    n98 = Equal?(x=w67, y=1.0) -> (x = y?=w56:bool)
    n99 = And(x=w56, y=w53) -> (x .and. y?=w22:bool)
    n100 = case shown="True" w72 {
      tunnel: "Back IR Object Distance" -> [w220 w236]
      tunnel: [w217 w229] -> w75
      tunnel: [w218 w228] -> w44
      tunnel: w30 -> [w219 w227]
      frame False {
        # "Converts hard value into index\nfor array"
        # "Divide by max voltage\nvalue to force\ndeceleration if object\nis too close"
        n101 = Divide(x=w220, y=80.0) -> (x/y=w225:dbl)
        n102 = Multiply(x=w225, y=100.0) -> (x*y=w226:dbl)
        n103 = Index Array(array=dbl[] [0.0, 0.5, 1.0, 1.5, 2.0, 2.5, 3.3, 3.0, 2.658255897, 2.408413052, 2.20488628, 2.035631323, 1.892484412, 1.769708211, 1.663148013, 1.569718295, 1.487077661, 1.413415986, 1.347310939, 1.287628787, 1.233454287, 1.184040141, 1.138769924, 1.097130449, 1.058690886, 1.023086768, 0.990007602, 0.959187169, 0.930395851, 0.903434503, 0.878129533, 0.854328896, 0.83189883, 0.81072117, 0.790691122, 0.771715412, 0.753710732, 0.736602435, 0.72032343, 0.704813241, 0.690017209, 0.675885801, 0.66237402, 0.64944089, 0.63704902, 0.625164212, 0.613755126, 0.602792986, 0.592251321, 0.582105738, 0.572333717, 0.562914438, 0.553828618, 0.545058374, 0.536587096, 0.528399334, 0.520480698, 0.51281777, 0.50539802, 0.498209735, 0.491241951, 0.484484395, 0.477927433, 0.471562015, 0.465379637, 0.459372298, 0.453532462, 0.447853023, 0.442327281, 0.436948907, 0.431711917, 0.426610656, 0.421639765, 0.416794173, 0.412069067, 0.407459883, 0.402962289, 0.398572167, 0.394285602, 0.39009887, 0.386008427, 0.382010895, 0.378103055, 0.374281838, 0.370544314, 0.366887686, 0.363309281, 0.359806547, 0.35637704, 0.353018422, 0.349728457, 0.346505002, 0.343346003, 0.340249491, 0.337213578, 0.334236453, 0.331316376, 0.328451676, 0.325640748, 0.32288205, 0.320174098] ("first row"), index=w226) -> (element=w224:dbl)
        n104 = Add(x=w224, y=w219) -> (x+y=w217:dbl)
        n105 = Divide(x=w217, y=3.3) -> (x/y=w218:dbl)
      }
      frame True {
        # "Forces a x1 multiplier\nessentially doing\nnothing to overall\nspeed."
        n106 = Divide(x=w236, y=80.0) -> (x/y=w234:dbl)
        n107 = Multiply(x=w234, y=100.0) -> (x*y=w235:dbl)
        n108 = Index Array(array=dbl[] [0.0, 0.5, 1.0, 1.5, 2.0, 2.5, 3.3, 3.0, 2.658255897, 2.408413052, 2.20488628, 2.035631323, 1.892484412, 1.769708211, 1.663148013, 1.569718295, 1.487077661, 1.413415986, 1.347310939, 1.287628787, 1.233454287, 1.184040141, 1.138769924, 1.097130449, 1.058690886, 1.023086768, 0.990007602, 0.959187169, 0.930395851, 0.903434503, 0.878129533, 0.854328896, 0.83189883, 0.81072117, 0.790691122, 0.771715412, 0.753710732, 0.736602435, 0.72032343, 0.704813241, 0.690017209, 0.675885801, 0.66237402, 0.64944089, 0.63704902, 0.625164212, 0.613755126, 0.602792986, 0.592251321, 0.582105738, 0.572333717, 0.562914438, 0.553828618, 0.545058374, 0.536587096, 0.528399334, 0.520480698, 0.51281777, 0.50539802, 0.498209735, 0.491241951, 0.484484395, 0.477927433, 0.471562015, 0.465379637, 0.459372298, 0.453532462, 0.447853023, 0.442327281, 0.436948907, 0.431711917, 0.426610656, 0.421639765, 0.416794173, 0.412069067, 0.407459883, 0.402962289, 0.398572167, 0.394285602, 0.39009887, 0.386008427, 0.382010895, 0.378103055, 0.374281838, 0.370544314, 0.366887686, 0.363309281, 0.359806547, 0.35637704, 0.353018422, 0.349728457, 0.346505002, 0.343346003, 0.340249491, 0.337213578, 0.334236453, 0.331316376, 0.328451676, 0.325640748, 0.32288205, 0.320174098] ("first row"), index=w235) -> (element=w233:dbl)
        n109 = Add(x=w233, y=w227) -> (x+y=w229:dbl)
        n110 = Divide(x=w229, y=w229) -> (x/y=w228:dbl)
      }
    }
    "Back IR Output voltage" <- w75
    n111 = And(x=w53, y=w54) -> (x .and. y?=w21:bool)
    n112 = Concatenate Strings(w84, ", other IP addresses = " ("string")) -> (w83:string)
    n113 = Not(x=w21) -> (.not. x?=w20:bool)
    n114 = Not(x=w22) -> (.not. x?=w23:bool)
    n115 = Not(x=w18) -> (.not. x?=w19:bool)
    n116 = Boolean To (0,1)(Boolean=w23) -> (0, 1=w51:i16)
    n117 = Or(x="Send", y=w87) -> (x .or. y?=w93:bool)
    n118 = Boolean To (0,1)(Boolean=w12) -> (0, 1=w141:i16)
    n119 = Boolean To (0,1)(Boolean=w19) -> (0, 1=w61:i16)
    n120 = Boolean To (0,1)(Boolean=w20) -> (0, 1=w64:i16)
    n121 = Boolean To (0,1)(Boolean=w15) -> (0, 1=w138:i16)
    n122 = Boolean To (0,1)(Boolean=w17) -> (0, 1=w142:i16)
    n123 = Multiply(x=w61, y=i16 10000) -> (x*y=w59:i16)
    n124 = Multiply(x=w51, y=i16 100) -> (x*y=w57:i16)
    n125 = Multiply(x=w64, y=i16 1000) -> (x*y=w58:i16)
    n126 = Multiply(x=w141, y=w132) -> (x*y=w140:i16)
    n127 = Multiply(x=w138, y=w137) -> (x*y=w139:i16)
    n128 = Multiply(x=w142, y=w136) -> (x*y=w143:i16)
    n129 = Compound Arithmetic op=ADD(w57, w58, w59, w143, w139, w140) -> (w135:i16)
    n130 = case shown="1" w135 {
      tunnel: ["Stop" "Hard Left" "Slight Forward" "Slight Left" "Hard Right" "Slight Forward" "Slight Right" "Forward" "Stop" "Hard Left" "Stop" "Hard Left" "Hard Right" "Stop" "Hard Right" "Stop" "Stop" "Hard Left" "Slight Forward" "Slight Left" "Hard Right" "Slight Forward" "Slight Right" "Slight Forward" "Stop" "Hard Left" "Stop" "Hard Left" "Stop" "Stop" "Stop" "Stop" "Stop" "Hard Left" "Slight Forward" "Slight Left" "Hard Right" "Slight Forward" "Slight Right" "Slight Forward" "Stop" "Stop" "Stop" "Stop" "Hard Right" "Stop" "Hard Right" "Stop" "Stop" "Stop" "Slight Forward" "Stop" "Stop" "Slight Forward" "Stop" "Slight Forward" "Stop" "Stop" "Stop" "Stop" "Stop" "Stop" "Stop" "Stop"] -> w154
      tunnel: [w327 w338 w349 w360 w371 w382 w393 w404 w413 w422 w433 w440 w452 w464 w473 w484 w493 w502 w512 w524 w535 w546 w553 w568 w577 w588 w597 w605 w619 w628 w637 w646 w655 w664 w675 w686 w697 w708 w719 w730 w741 w750 w759 w768 w777 w785 w797 w808 w817 w826 w835 w846 w855 w864 w875 w881 w895 w904 w914 w922 w931 w938 w950 w958] -> w131
      tunnel: [w325 w335 w345 w356 w368 w378 w389 w401 w412 w421 w432 w441 w453 w463 w472 w483 w492 w501 w511 w523 w534 w545 w555 w567 w578 w587 w598 w606 w618 w627 w636 w645 w654 w663 w674 w685 w696 w707 w718 w729 w740 w749 w758 w767 w776 w786 w796 w807 w816 w825 w834 w845 w854 w863 w874 w882 w894 w903 w913 w921 w930 w939 w949 w957] -> w112
      tunnel: [w326 w334 w346 w357 w367 w379 w390 w400 w414 w423 w434 w439 w454 w465 w474 w485 w494 w503 w513 w525 w536 w547 w554 w569 w576 w589 w596 w604 w620 w629 w638 w647 w656 w665 w676 w687 w698 w709 w720 w731 w742 w751 w760 w769 w778 w784 w798 w809 w818 w827 w836 w847 w856 w865 w876 w880 w896 w905 w909 w923 w932 w937 w948 w959] -> w114
      tunnel: ["Place robot on line!" "" "" "" "" "" "" "" "Warning! Obstruction ahead! Place robot on the line!" "Warning! Obstruction Ahead!" "Warning! Obstruction ahead! Stopping!" "Warning! Obstruction Ahead! Evasive action!" "Warning! Obstruction Ahead!" "Warning! Obstruction ahead! Stopping!" "Warning! Obstruction Ahead! Evasive Action!" "Warning! Obstruction Ahead! Stopping!" "Warning! Obstruction to the Right! Place robot on line!" "Warning! Obstruction to the Right! Repositioning and stopping!" "Warning! Obstruction to the Right! Slowing!" "Warning! Obstruction to the Right! Slowing!" "Warning! Obstruction to the Right!" "Warning! Obstruction to the Right! Slowing!" "Warning! Obstruction to the Right! Slowing!" "Warning! Obstruction to the Right! Slowing!" "Warning! Obstruction to the Right! Obstruction Ahead! Place robot on line!" "Warning! Obstruction to the Right! Obstruction Ahead! " "Warning! Obstruction to the Right! Obstruction Ahead! Stopping!" "Warning! Obstruction to the Right! Obstruction Ahead! Evasive Action!" "Warning! Obstruction to the Right! Obstruction Ahead! Repositioning and stopping!" "Warning! Obstruction to the Right! Obstruction Ahead! Stopping!" "Warning! Obstruction to the Right! Obstruction Ahead! Repositioning and stopping!" "Warning! Obstruction to the Right! Obstruction Ahead! Stopping!" "Warning! Obstruction to the Left! Obstruction Ahead! Place robot on line!" "Warning! Obstruction to the Left! Repositioning and stopping!" "Warning! Obstruction to the Left! Slowing!" "Warning! Obstruction to the Left! Slowing!" "Warning! Obstruction to the Left!" "Warning! Obstruction to the Left! Slowing!" "Warning! Obstruction to the Left! Slowing" "Warning! Obstruction to the Left! Slowing!" "Warning! Obstruction to the Left! Obstruction Ahead! Place robot on line!" "Warning! Obstruction to the Left! Obstruction Ahead!" "Warning! Obstruction to the Left! Obstruction Ahead!" "Warning! Obstruction to the Left! Obstruction Ahead!" "Warning! Obstruction to the Left! Obstruction Ahead!" "Warning! Obstruction to the Left! Obstruction Ahead!" "Warning! Obstruction to the Left! Obstruction Ahead!" "Warning! Obstruction to the Left! Obstruction Ahead! Stopping!" "Warning! Obstruction to the Left! Obstruction to the Right! Place robot on line!" "Warning! Obstruction to the Left! Obstruction to the Right! Stopping!" "Warning! Obstruction to the Left! Obstruction to the Right! Slowing!" "Warning! Obstruction to the Left! Obstruction to the Right! Stopping!" "Warning! Obstruction to the Left! Obstruction to the Right! Stopping!" "Warning! Obstruction to the Left! Obstruction to the Right! Slowing!" "Warning! Obstruction to the Left! Obstruction to the Right! Stopping!" "Warning! Obstruction to the Left! Obstruction to the Right! Slowing!" "Warning! Total Obstruction! Stopping!" "Warning! Total Obstruction! Stopping!" "Warning! Total Obstruction! Stopping!" "Warning! Total Obstruction! Stopping!" "Warning! Total Obstruction! Stopping!" "Warning! Total Obstruction! Stopping!" "Warning! Total Obstruction! Stopping!" "Warning! Total Obstruction! Stopping!"] -> w43
      tunnel: [TRUE FALSE FALSE FALSE FALSE FALSE FALSE FALSE TRUE TRUE TRUE TRUE TRUE TRUE TRUE TRUE TRUE TRUE TRUE TRUE TRUE TRUE TRUE TRUE TRUE TRUE TRUE TRUE TRUE TRUE TRUE TRUE TRUE TRUE TRUE TRUE TRUE TRUE TRUE TRUE TRUE TRUE TRUE TRUE TRUE TRUE TRUE TRUE TRUE TRUE TRUE TRUE TRUE TRUE TRUE TRUE TRUE TRUE TRUE TRUE TRUE TRUE TRUE TRUE] -> w40
      tunnel: [w322 w331 w342 w353 w364 w375 w386 w397 w408 w417 w428 w437 w448 w459 w468 w479 w488 w497 w508 w519 w530 w541 w552 w563 w574 w583 w594 w603 w614 w623 w632 w641 w650 w659 w670 w681 w692 w703 w714 w725 w736 w745 w754 w763 w772 w783 w792 w803 w812 w821 w830 w841 w850 w859 w870 w879 w890 w899 w908 w917 w926 w935 w944 w953] -> w42
      frame 0, Default {
        w325 = 0.0  # Right Motor Stopped
        w326 = 0.0  # Left Motor Stopped
        n131 = Add(x=w326, y=w325) -> (x+y=w329:dbl)
        n132 = Divide(x=w329, y=2.0) -> (x/y=w327:dbl)
        n133 = First Call?() -> (First Call?: T/F=w322:bool)
      }
      frame 1 {
        w336 = -1.0  # Right Motor Forwards
        w334 = -1.0  # Left Motor Backwards
        n134 = Multiply(x=w336, y=-1.0) -> (x*y=w335:dbl)
        n135 = Add(x=w334, y=w335) -> (x+y=w340:dbl)
        n136 = Divide(x=w340, y=2.0) -> (x/y=w338:dbl)
        n137 = First Call?() -> (First Call?: T/F=w331:bool)
      }
      frame 5 {
        w347 = -0.5  # Right Motor Forwards
        w346 = 0.5  # Left Motor Forwards
        # "Case 5 pressumes potential break\nin line and continues as normal.\nMotor coefficient changed to 0.5\nincase robot isn't on the line."
        n138 = Multiply(x=w347, y=-1.0) -> (x*y=w345:dbl)
        n139 = Add(x=w346, y=w345) -> (x+y=w351:dbl)
        n140 = Divide(x=w351, y=2.0) -> (x/y=w349:dbl)
        n141 = First Call?() -> (First Call?: T/F=w342:bool)
      }
      frame 6 {
        w358 = -1.0  # Right Motor Forwards
        w357 = 0.5  # Left Motor Forwards
        # "Left motor slows for gradual\nturning. Left motor coefficient\nchanges to 0.5."
        n142 = Multiply(x=w358, y=-1.0) -> (x*y=w356:dbl)
        n143 = Add(x=w357, y=w356) -> (x+y=w362:dbl)
        n144 = Divide(x=w362, y=2.0) -> (x/y=w360:dbl)
        n145 = First Call?() -> (First Call?: T/F=w353:bool)
      }
      frame 10 {
        w369 = 1.0  # Right Motor Backwards
        w367 = 1.0  # Left Motor Forwards
        n146 = Multiply(x=w369, y=-1.0) -> (x*y=w368:dbl)
        n147 = Add(x=w367, y=w368) -> (x+y=w373:dbl)
        n148 = Divide(x=w373, y=2.0) -> (x/y=w371:dbl)
        n149 = First Call?() -> (First Call?: T/F=w364:bool)
      }
      frame 11 {
        w380 = -0.5  # Right Motor Forwards
        w379 = 0.5  # Left Motor Forwards
        # "Case 11 presumes that line breaks in the \nmiddle and keeps going forward. Motor\ncoefficient changed to 0.5 incase it is\nnot on the line."
        n150 = Multiply(x=w380, y=-1.0) -> (x*y=w378:dbl)
        n151 = Add(x=w379, y=w378) -> (x+y=w384:dbl)
        n152 = Divide(x=w384, y=2.0) -> (x/y=w382:dbl)
        n153 = First Call?() -> (First Call?: T/F=w375:bool)
      }
      frame 15 {
        w391 = -0.5  # Right Motor Forwards
        w390 = 1.0  # Left Motor Forwards
        # "Right motor slows for gradual\nturning. Right motor coefficient\nchanges to 0.5."
        n154 = Multiply(x=w391, y=-1.0) -> (x*y=w389:dbl)
        n155 = Add(x=w390, y=w389) -> (x+y=w395:dbl)
        n156 = Divide(x=w395, y=2.0) -> (x/y=w393:dbl)
        n157 = First Call?() -> (First Call?: T/F=w386:bool)
      }
      frame 16 {
        w402 = -1.0  # Right Motor Forwards
        w400 = 1.0  # Left Motor Forwards
        n158 = Multiply(x=w402, y=-1.0) -> (x*y=w401:dbl)
        n159 = Add(x=w400, y=w401) -> (x+y=w406:dbl)
        n160 = Divide(x=w406, y=2.0) -> (x/y=w404:dbl)
        n161 = First Call?() -> (First Call?: T/F=w397:bool)
      }
      frame 100 {
        w412 = 0.0  # Right Motor Stopped
        w414 = 0.0  # Left Motor Stopped
        n162 = Add(x=w414, y=w412) -> (x+y=w416:dbl)
        n163 = Divide(x=w416, y=2.0) -> (x/y=w413:dbl)
        n164 = First Call?() -> (First Call?: T/F=w408:bool)
      }
      frame 101 {
        w424 = -1.0  # Right Motor Forwards
        w423 = -1.0  # Left Motor Backwards
        n165 = Multiply(x=w424, y=-1.0) -> (x*y=w421:dbl)
        n166 = Add(x=w423, y=w421) -> (x+y=w427:dbl)
        n167 = Divide(x=w427, y=2.0) -> (x/y=w422:dbl)
        n168 = First Call?() -> (First Call?: T/F=w417:bool)
      }
      frame 105 {
        w432 = 0.0  # Right Motor Stopped
        w434 = 0.0  # Left Motor Stopped
        n169 = Add(x=w434, y=w432) -> (x+y=w436:dbl)
        n170 = Divide(x=w436, y=2.0) -> (x/y=w433:dbl)
        n171 = First Call?() -> (First Call?: T/F=w428:bool)
      }
      frame 106 {
        w443 = -1.0  # Right Motor Forwards
        w439 = -1.0  # Left Motor Backwards
        n172 = Multiply(x=w443, y=-1.0) -> (x*y=w441:dbl)
        n173 = Add(x=w439, y=w441) -> (x+y=w446:dbl)
        n174 = Divide(x=w446, y=2.0) -> (x/y=w440:dbl)
        n175 = First Call?() -> (First Call?: T/F=w437:bool)
      }
      frame 110 {
        w455 = 1.0  # Right Motor Backwards
        w454 = 1.0  # Left Motor Forwards
        n176 = Multiply(x=w455, y=-1.0) -> (x*y=w453:dbl)
        n177 = Add(x=w454, y=w453) -> (x+y=w458:dbl)
        n178 = Divide(x=w458, y=2.0) -> (x/y=w452:dbl)
        n179 = First Call?() -> (First Call?: T/F=w448:bool)
      }
      frame 111 {
        w463 = 0.0  # Right Motor Stopped
        w465 = 0.0  # Left Motor Stopped
        n180 = Add(x=w465, y=w463) -> (x+y=w467:dbl)
        n181 = Divide(x=w467, y=2.0) -> (x/y=w464:dbl)
        n182 = First Call?() -> (First Call?: T/F=w459:bool)
      }
      frame 115 {
        w475 = 1.0  # Right Motor Backwards
        w474 = 1.0  # Left Motor Forwards
        n183 = Multiply(x=w475, y=-1.0) -> (x*y=w472:dbl)
        n184 = Add(x=w474, y=w472) -> (x+y=w478:dbl)
        n185 = Divide(x=w478, y=2.0) -> (x/y=w473:dbl)
        n186 = First Call?() -> (First Call?: T/F=w468:bool)
      }
      frame 116 {
        w483 = 0.0  # Right Motor Stopped
        w485 = 0.0  # Left Motor Stopped
        n187 = Add(x=w485, y=w483) -> (x+y=w487:dbl)
        n188 = Divide(x=w487, y=2.0) -> (x/y=w484:dbl)
        n189 = First Call?() -> (First Call?: T/F=w479:bool)
      }
      frame 1000 {
        w492 = 0.0  # Right Motor Stopped
        w494 = 0.0  # Left Motor Stopped
        n190 = Add(x=w494, y=w492) -> (x+y=w496:dbl)
        n191 = Divide(x=w496, y=2.0) -> (x/y=w493:dbl)
        n192 = First Call?() -> (First Call?: T/F=w488:bool)
      }
      frame 1001 {
        w504 = -1.0  # Right Motor Forwards
        w503 = -1.0  # Left Motor Backwards
        n193 = Multiply(x=w504, y=-1.0) -> (x*y=w501:dbl)
        n194 = Add(x=w503, y=w501) -> (x+y=w507:dbl)
        n195 = Divide(x=w507, y=2.0) -> (x/y=w502:dbl)
        n196 = First Call?() -> (First Call?: T/F=w497:bool)
      }
      frame 1005 {
        w515 = -0.25  # Right Motor Forwards
        w513 = 0.25  # Left Motor Forwards
        n197 = Multiply(x=w515, y=-1.0) -> (x*y=w511:dbl)
        n198 = Add(x=w513, y=w511) -> (x+y=w518:dbl)
        n199 = Divide(x=w518, y=2.0) -> (x/y=w512:dbl)
        n200 = First Call?() -> (First Call?: T/F=w508:bool)
      }
      frame 1006 {
        w526 = -0.5  # Right Motor Forwards
        w525 = 0.25  # Left Motor Forwards
        n201 = Multiply(x=w526, y=-1.0) -> (x*y=w523:dbl)
        n202 = Add(x=w525, y=w523) -> (x+y=w529:dbl)
        n203 = Divide(x=w529, y=2.0) -> (x/y=w524:dbl)
        n204 = First Call?() -> (First Call?: T/F=w519:bool)
      }
      frame 1010 {
        w537 = 1.0  # Right Motor Backwards
        w536 = 1.0  # Left Motor Forwards
        n205 = Multiply(x=w537, y=-1.0) -> (x*y=w534:dbl)
        n206 = Add(x=w536, y=w534) -> (x+y=w540:dbl)
        n207 = Divide(x=w540, y=2.0) -> (x/y=w535:dbl)
        n208 = First Call?() -> (First Call?: T/F=w530:bool)
      }
      frame 1011 {
        w548 = -0.25  # Right Motor Forwards
        w547 = 0.25  # Left Motor Forwards
        n209 = Multiply(x=w548, y=-1.0) -> (x*y=w545:dbl)
        n210 = Add(x=w547, y=w545) -> (x+y=w551:dbl)
        n211 = Divide(x=w551, y=2.0) -> (x/y=w546:dbl)
        n212 = First Call?() -> (First Call?: T/F=w541:bool)
      }
      frame 1015 {
        w559 = -0.25  # Right Motor Forwards
        w554 = 0.5  # Left Motor Forwards
        n213 = Multiply(x=w559, y=-1.0) -> (x*y=w555:dbl)
        n214 = Add(x=w554, y=w555) -> (x+y=w562:dbl)
        n215 = Divide(x=w562, y=2.0) -> (x/y=w553:dbl)
        n216 = First Call?() -> (First Call?: T/F=w552:bool)
      }
      frame 1016 {
        w570 = -0.25  # Right Motor Forwards
        w569 = 0.25  # Left Motor Forwards
        n217 = Multiply(x=w570, y=-1.0) -> (x*y=w567:dbl)
        n218 = Add(x=w569, y=w567) -> (x+y=w573:dbl)
        n219 = Divide(x=w573, y=2.0) -> (x/y=w568:dbl)
        n220 = First Call?() -> (First Call?: T/F=w563:bool)
      }
      frame 1100 {
        w578 = 0.0  # Right Motor Stopped
        w576 = 0.0  # Left Motor Stopped
        n221 = Add(x=w576, y=w578) -> (x+y=w582:dbl)
        n222 = Divide(x=w582, y=2.0) -> (x/y=w577:dbl)
        n223 = First Call?() -> (First Call?: T/F=w574:bool)
      }
      frame 1101 {
        w590 = -1.0  # Right Motor Forwards
        w589 = -1.0  # Left Motor Backwards
        n224 = Multiply(x=w590, y=-1.0) -> (x*y=w587:dbl)
        n225 = Add(x=w589, y=w587) -> (x+y=w593:dbl)
        n226 = Divide(x=w593, y=2.0) -> (x/y=w588:dbl)
        n227 = First Call?() -> (First Call?: T/F=w583:bool)
      }
      frame 1105 {
        w598 = 0.0  # Right Motor Stopped
        w596 = 0.0  # Left Motor Stopped
        n228 = Add(x=w596, y=w598) -> (x+y=w602:dbl)
        n229 = Divide(x=w602, y=2.0) -> (x/y=w597:dbl)
        n230 = First Call?() -> (First Call?: T/F=w594:bool)
      }
      frame 1106 {
        w610 = -1.0  # Right Motor Forwards
        w604 = -1.0  # Left Motor Backwards
        n231 = Multiply(x=w610, y=-1.0) -> (x*y=w606:dbl)
        n232 = Add(x=w604, y=w606) -> (x+y=w613:dbl)
        n233 = Divide(x=w613, y=2.0) -> (x/y=w605:dbl)
        n234 = First Call?() -> (First Call?: T/F=w603:bool)
      }
      frame 1110 {
        w618 = 0.0  # Right Motor Stopped
        w620 = 0.0  # Left Motor Stopped
        n235 = Add(x=w620, y=w618) -> (x+y=w622:dbl)
        n236 = Divide(x=w622, y=2.0) -> (x/y=w619:dbl)
        n237 = First Call?() -> (First Call?: T/F=w614:bool)
      }
      frame 1111 {
        w627 = 0.0  # Right Motor Stopped
        w629 = 0.0  # Left Motor Stopped
        n238 = Add(x=w629, y=w627) -> (x+y=w631:dbl)
        n239 = Divide(x=w631, y=2.0) -> (x/y=w628:dbl)
        n240 = First Call?() -> (First Call?: T/F=w623:bool)
      }
      frame 1115 {
        w636 = 0.0  # Right Motor Stopped
        w638 = 0.0  # Left Motor Stopped
        n241 = Add(x=w638, y=w636) -> (x+y=w640:dbl)
        n242 = Divide(x=w640, y=2.0) -> (x/y=w637:dbl)
        n243 = First Call?() -> (First Call?: T/F=w632:bool)
      }
      frame 1116 {
        w645 = 0.0  # Right Motor Stopped
        w647 = 0.0  # Left Motor Stopped
        n244 = Add(x=w647, y=w645) -> (x+y=w649:dbl)
        n245 = Divide(x=w649, y=2.0) -> (x/y=w646:dbl)
        n246 = First Call?() -> (First Call?: T/F=w641:bool)
      }
      frame 10000 {
        w654 = 0.0  # Right Motor Stopped
        w656 = 0.0  # Left Motor Stopped
        # "Stop"
        n247 = Add(x=w656, y=w654) -> (x+y=w658:dbl)
        n248 = Divide(x=w658, y=2.0) -> (x/y=w655:dbl)
        n249 = First Call?() -> (First Call?: T/F=w650:bool)
      }
      frame 10001 {
        w666 = -1.0  # Right Motor Forwards
        w665 = -1.0  # Left Motor Backwards
        n250 = Multiply(x=w666, y=-1.0) -> (x*y=w663:dbl)
        n251 = Add(x=w665, y=w663) -> (x+y=w669:dbl)
        n252 = Divide(x=w669, y=2.0) -> (x/y=w664:dbl)
        n253 = First Call?() -> (First Call?: T/F=w659:bool)
      }
      frame 10005 {
        w677 = -0.25  # Right Motor Forwards
        w676 = 0.25  # Left Motor Forwards
        n254 = Multiply(x=w677, y=-1.0) -> (x*y=w674:dbl)
        n255 = Add(x=w676, y=w674) -> (x+y=w680:dbl)
        n256 = Divide(x=w680, y=2.0) -> (x/y=w675:dbl)
        n257 = First Call?() -> (First Call?: T/F=w670:bool)
      }
      frame 10006 {
        w688 = -0.5  # Right Motor Forwards
        w687 = 0.25  # Left Motor Forwards
        n258 = Multiply(x=w688, y=-1.0) -> (x*y=w685:dbl)
        n259 = Add(x=w687, y=w685) -> (x+y=w691:dbl)
        n260 = Divide(x=w691, y=2.0) -> (x/y=w686:dbl)
        n261 = First Call?() -> (First Call?: T/F=w681:bool)
      }
      frame 10010 {
        w699 = 1.0  # Right Motor Backwards
        w698 = 1.0  # Left Motor Forwards
        n262 = Multiply(x=w699, y=-1.0) -> (x*y=w696:dbl)
        n263 = Add(x=w698, y=w696) -> (x+y=w702:dbl)
        n264 = Divide(x=w702, y=2.0) -> (x/y=w697:dbl)
        n265 = First Call?() -> (First Call?: T/F=w692:bool)
      }
      frame 10011 {
        w710 = -0.25  # Right Motor Forwards
        w709 = 0.25  # Left Motor Forwards
        n266 = Multiply(x=w710, y=-1.0) -> (x*y=w707:dbl)
        n267 = Add(x=w709, y=w707) -> (x+y=w713:dbl)
        n268 = Divide(x=w713, y=2.0) -> (x/y=w708:dbl)
        n269 = First Call?() -> (First Call?: T/F=w703:bool)
      }
      frame 10015 {
        w721 = -0.25  # Right Motor Forwards
        w720 = 0.5  # Left Motor Forwards
        n270 = Multiply(x=w721, y=-1.0) -> (x*y=w718:dbl)
        n271 = Add(x=w720, y=w718) -> (x+y=w724:dbl)
        n272 = Divide(x=w724, y=2.0) -> (x/y=w719:dbl)
        n273 = First Call?() -> (First Call?: T/F=w714:bool)
      }
      frame 10016 {
        w732 = -0.25  # Right Motor Forwards
        w731 = 0.25  # Left Motor Forwards
        n274 = Multiply(x=w732, y=-1.0) -> (x*y=w729:dbl)
        n275 = Add(x=w731, y=w729) -> (x+y=w735:dbl)
        n276 = Divide(x=w735, y=2.0) -> (x/y=w730:dbl)
        n277 = First Call?() -> (First Call?: T/F=w725:bool)
      }
      frame 10100 {
        w740 = 0.0  # Right Motor Stopped
        w742 = 0.0  # Left Motor Stopped
        # "Stop"
        n278 = Add(x=w742, y=w740) -> (x+y=w744:dbl)
        n279 = Divide(x=w744, y=2.0) -> (x/y=w741:dbl)
        n280 = First Call?() -> (First Call?: T/F=w736:bool)
      }
      frame 10101 {
        w749 = 0.0  # Right Motor Stopped
        w751 = 0.0  # Left Motor Stopped
        n281 = Add(x=w751, y=w749) -> (x+y=w753:dbl)
        n282 = Divide(x=w753, y=2.0) -> (x/y=w750:dbl)
        n283 = First Call?() -> (First Call?: T/F=w745:bool)
      }
      frame 10105 {
        w758 = 0.0  # Right Motor Stopped
        w760 = 0.0  # Left Motor Stopped
        n284 = Add(x=w760, y=w758) -> (x+y=w762:dbl)
        n285 = Divide(x=w762, y=2.0) -> (x/y=w759:dbl)
        n286 = First Call?() -> (First Call?: T/F=w754:bool)
      }
      frame 10106 {
        w767 = 0.0  # Right Motor Stopped
        w769 = 0.0  # Left Motor Stopped
        n287 = Add(x=w769, y=w767) -> (x+y=w771:dbl)
        n288 = Divide(x=w771, y=2.0) -> (x/y=w768:dbl)
        n289 = First Call?() -> (First Call?: T/F=w763:bool)
      }
      frame 10110 {
        w779 = 1.0  # Right Motor Backwards
        w778 = 1.0  # Left Motor Forwards
        n290 = Multiply(x=w779, y=-1.0) -> (x*y=w776:dbl)
        n291 = Add(x=w778, y=w776) -> (x+y=w782:dbl)
        n292 = Divide(x=w782, y=2.0) -> (x/y=w777:dbl)
        n293 = First Call?() -> (First Call?: T/F=w772:bool)
      }
      frame 10111 {
        w786 = 0.0  # Right Motor Stopped
        w784 = 0.0  # Left Motor Stopped
        n294 = Add(x=w784, y=w786) -> (x+y=w791:dbl)
        n295 = Divide(x=w791, y=2.0) -> (x/y=w785:dbl)
        n296 = First Call?() -> (First Call?: T/F=w783:bool)
      }
      frame 10115 {
        w799 = 1.0  # Right Motor Backwards
        w798 = 1.0  # Left Motor Forwards
        n297 = Multiply(x=w799, y=-1.0) -> (x*y=w796:dbl)
        n298 = Add(x=w798, y=w796) -> (x+y=w802:dbl)
        n299 = Divide(x=w802, y=2.0) -> (x/y=w797:dbl)
        n300 = First Call?() -> (First Call?: T/F=w792:bool)
      }
      frame 10116 {
        w807 = 0.0  # Right Motor Stopped
        w809 = 0.0  # Left Motor Stopped
        n301 = Add(x=w809, y=w807) -> (x+y=w811:dbl)
        n302 = Divide(x=w811, y=2.0) -> (x/y=w808:dbl)
        n303 = First Call?() -> (First Call?: T/F=w803:bool)
      }
      frame 11000 {
        w816 = 0.0  # Right Motor Stopped
        w818 = 0.0  # Left Motor Stopped
        # "Stop"
        n304 = Add(x=w818, y=w816) -> (x+y=w820:dbl)
        n305 = Divide(x=w820, y=2.0) -> (x/y=w817:dbl)
        n306 = First Call?() -> (First Call?: T/F=w812:bool)
      }
      frame 11001 {
        w825 = 0.0  # Right Motor Stopped
        w827 = 0.0  # Left Motor Stopped
        n307 = Add(x=w827, y=w825) -> (x+y=w829:dbl)
        n308 = Divide(x=w829, y=2.0) -> (x/y=w826:dbl)
        n309 = First Call?() -> (First Call?: T/F=w821:bool)
      }
      frame 11005 {
        w837 = -0.25  # Right Motor Forwards
        w836 = 0.25  # Left Motor Forwards
        n310 = Multiply(x=w837, y=-1.0) -> (x*y=w834:dbl)
        n311 = Add(x=w836, y=w834) -> (x+y=w840:dbl)
        n312 = Divide(x=w840, y=2.0) -> (x/y=w835:dbl)
        n313 = First Call?() -> (First Call?: T/F=w830:bool)
      }
      frame 11006 {
        w845 = 0.0  # Right Motor Stopped
        w847 = 0.0  # Left Motor Stopped
        n314 = Add(x=w847, y=w845) -> (x+y=w849:dbl)
        n315 = Divide(x=w849, y=2.0) -> (x/y=w846:dbl)
        n316 = First Call?() -> (First Call?: T/F=w841:bool)
      }
      frame 11010 {
        w854 = 0.0  # Right Motor Stopped
        w856 = 0.0  # Left Motor Stopped
        n317 = Add(x=w856, y=w854) -> (x+y=w858:dbl)
        n318 = Divide(x=w858, y=2.0) -> (x/y=w855:dbl)
        n319 = First Call?() -> (First Call?: T/F=w850:bool)
      }
      frame 11011 {
        w866 = -0.25  # Right Motor Forwards
        w865 = 0.25  # Left Motor Forwards
        n320 = Multiply(x=w866, y=-1.0) -> (x*y=w863:dbl)
        n321 = Add(x=w865, y=w863) -> (x+y=w869:dbl)
        n322 = Divide(x=w869, y=2.0) -> (x/y=w864:dbl)
        n323 = First Call?() -> (First Call?: T/F=w859:bool)
      }
      frame 11015 {
        w874 = 0.0  # Right Motor Stopped
        w876 = 0.0  # Left Motor Stopped
        n324 = Add(x=w876, y=w874) -> (x+y=w878:dbl)
        n325 = Divide(x=w878, y=2.0) -> (x/y=w875:dbl)
        n326 = First Call?() -> (First Call?: T/F=w870:bool)
      }
      frame 11016 {
        w886 = -0.25  # Right Motor Forwards
        w880 = 0.25  # Left Motor Forwards
        n327 = Multiply(x=w886, y=-1.0) -> (x*y=w882:dbl)
        n328 = Add(x=w880, y=w882) -> (x+y=w889:dbl)
        n329 = Divide(x=w889, y=2.0) -> (x/y=w881:dbl)
        n330 = First Call?() -> (First Call?: T/F=w879:bool)
      }
      frame 11100 {
        w894 = 0.0  # Right Motor Stopped
        w896 = 0.0  # Left Motor Stopped
        # "Stop"
        n331 = Add(x=w896, y=w894) -> (x+y=w898:dbl)
        n332 = Divide(x=w898, y=2.0) -> (x/y=w895:dbl)
        n333 = First Call?() -> (First Call?: T/F=w890:bool)
      }
      frame 11101 {
        w903 = 0.0  # Right Motor Stopped
        w905 = 0.0  # Left Motor Stopped
        n334 = Add(x=w905, y=w903) -> (x+y=w907:dbl)
        n335 = Divide(x=w907, y=2.0) -> (x/y=w904:dbl)
        n336 = First Call?() -> (First Call?: T/F=w899:bool)
      }
      frame 11105 {
        w913 = 0.0  # Right Motor Stopped
        w909 = 0.0  # Left Motor Stopped
        n337 = Add(x=w909, y=w913) -> (x+y=w916:dbl)
        n338 = Divide(x=w916, y=2.0) -> (x/y=w914:dbl)
        n339 = First Call?() -> (First Call?: T/F=w908:bool)
      }
      frame 11106 {
        w921 = 0.0  # Right Motor Stopped
        w923 = 0.0  # Left Motor Stopped
        n340 = Add(x=w923, y=w921) -> (x+y=w925:dbl)
        n341 = Divide(x=w925, y=2.0) -> (x/y=w922:dbl)
        n342 = First Call?() -> (First Call?: T/F=w917:bool)
      }
      frame 11110 {
        w930 = 0.0  # Right Motor Stopped
        w932 = 0.0  # Left Motor Stopped
        n343 = Add(x=w932, y=w930) -> (x+y=w934:dbl)
        n344 = Divide(x=w934, y=2.0) -> (x/y=w931:dbl)
        n345 = First Call?() -> (First Call?: T/F=w926:bool)
      }
      frame 11111 {
        w939 = 0.0  # Right Motor Stopped
        w937 = 0.0  # Left Motor Stopped
        n346 = Add(x=w937, y=w939) -> (x+y=w943:dbl)
        n347 = Divide(x=w943, y=2.0) -> (x/y=w938:dbl)
        n348 = First Call?() -> (First Call?: T/F=w935:bool)
      }
      frame 11115 {
        w949 = 0.0  # Right Motor Stopped
        w948 = 0.0  # Left Motor Stopped
        n349 = Add(x=w948, y=w949) -> (x+y=w952:dbl)
        n350 = Divide(x=w952, y=2.0) -> (x/y=w950:dbl)
        n351 = First Call?() -> (First Call?: T/F=w944:bool)
      }
      frame 11116 {
        w957 = 0.0  # Right Motor Stopped
        w959 = 0.0  # Left Motor Stopped
        n352 = Add(x=w959, y=w957) -> (x+y=w961:dbl)
        n353 = Divide(x=w961, y=2.0) -> (x/y=w958:dbl)
        n354 = First Call?() -> (First Call?: T/F=w953:bool)
      }
    }
    "Direction" <- w154
    "Warning Message" <- w43
    n355 = Concatenate Strings("Data = " ("string"), w78, ",  current IP address = " ("string")) -> (w86:string)
    n356 = Concatenate Strings(w86, w83, w81, "Message") -> (w88:string)
    "String" <- w88
    n357 = case shown="True" w93 {
      tunnel: "Subject" -> [_ w260]
      tunnel: "Recipients" -> [_ w259]
      tunnel: w88 -> [_ w258]
      frame False {
      }
      frame True {
        n358 = call "Send Email"("Message"=w258, "Subject"=w260, "Recipients"=w259) -> ("error out"=→"error out":errorcluster)  [unwired: 8 in]
      }
    }
    n359 = Divide(x="% Power", y=100.0) -> (x/y=w144:dbl)
    n360 = Multiply(x=w151, y=3.141592653589793) -> (x*y=w148:dbl)
    n361 = Divide(x=w153, y=w152) -> (x/y=w149:dbl)
    n362 = Multiply(x=w149, y=w148) -> (x*y=w147:dbl)
    n363 = Multiply(x=w144, y=w147) -> (x*y=w28:dbl)
    n364 = Multiply(x=w28, y=w131) -> (x*y=→"Speedometer (m/s)":dbl)
    n365 = Multiply(x=w28, y=w112) -> (x*y=→"Right Motor Speedometer (m/s)":dbl)
    n366 = And(x=w42, y=w40) -> (x .and. y?=w41:bool)
    n367 = Multiply(x=w28, y=w114) -> (x*y=→"Left Motor Speedometer (m/s)":dbl)
    n368 = case shown="True" w41 {
      tunnel: w43 -> [w164 w165]
      frame False {
        "String 2" <- w164
      }
      frame True {
        w167 = ""
        w168 = 0 items=["SVSFDefault"=0, "SVSFlagsAsync"=1, "SVSFPurgeBeforeSpeak"=2, "SVSFIsFilename"=4, "SVSFIsXML"=8, "SVSFIsNotXML"=16, "SVSFPersistXML"=32, "SVSFNLPSpeakPunc, SVSFNLPMask"=64, "SVSFVoiceMask"=127, "SVSFUnusedFlags"=-128] ("Flags")
        n369 = Automation Open(Automation Refnum="SpeechLib.ISpeechVoice") -> (Automation Refnum=w185:refnum<k7>, error out=w179:errorcluster)  [unwired: 1 in, 2 out]
        n370 = invoke class="ISpeechVoice" method="GetVoices"(reference=w185, error in=w179, "RequiredAttributes"=w167, "OptionalAttributes"=w167) -> (reference out=w184:refnum<k7>, error out=w178:errorcluster, "GetVoices"=w177:refnum<k7>)  [unwired: 1 in, 2 out]
        n371 = for {
          N: 3 -> [_]
          tunnel: [w193] -> w171
          tunnel: w178 -> [w190]
          tunnel: w177 -> [w189]
          tunnel: [w188] -> w176
          tunnel: [w187] -> w175 mode=indexing
          i -> [w192]
          n372 = invoke class="ISpeechObjectTokens" method="Item"(reference=w189, error in=w190, "Index"=w192) -> (reference out=w188:refnum<k7>, error out=w193:errorcluster, "Item"=w194:refnum<k7>)  [unwired: 1 in, 1 out]
          n373 = invoke class="ISpeechObjectToken" method="GetDescription"(reference=w194) -> (reference out=w191:refnum<k7>, "GetDescription"=w187:string)  [unwired: 3 in, 2 out]
          n374 = Close Reference(reference=w191) -> ()  [unwired: 1 in, 1 out]
        }
        n375 = invoke class="ISpeechObjectTokens" method="Item"(reference=w176, error in=w171, "Index"="CHOOSE A VOICE:") -> (reference out=w172:refnum<k7>, error out=w170:errorcluster, "Item"=w180:refnum<k7>)  [unwired: 1 in, 1 out]
        n376 = property on="CHOOSE A VOICE:" class="Ring (strict)"("Strings []"=w175) -> ()  [unwired: 2 in, 2 out]
        n377 = Close Reference(reference=w172, error in (no error)=w170) -> (error out=w169:errorcluster)
        n378 = property class="ISpeechVoice"(reference=w184, error in=w169, "Voice"=w180) -> (reference out=w183:refnum<k7>, error out=w182:errorcluster)
        n379 = invoke class="ISpeechVoice" method="Speak"(reference=w183, error in=w182, "Text"=w165, "Flags"=w168) -> (reference out=→"SpeechLib.ISpeechVoice 2":refnum<k7>, error out=w173:errorcluster)  [unwired: 1 in, 3 out]
        n380 = call <vilib>:"Simple Error Handler.vi"("error in (no error)"=w173) -> ()  [unwired: 1 in, 8 out]
      }
    }
    n381 = Not Equal?(x=w44, y=1.0) -> (x != y?=w45:bool)
    n382 = Or(x=w45, y=w40) -> (x .or. y?=→"Caution":bool)
  }
  n383 = call <vilib>:"IMAQdx Close Camera.vi"("Session In"=w1) -> ()  [unwired: 10 in, 1 out]
